vi "Main.vi"() -> ()   [LabVIEW 2013]
doc: "Use this template to build a producer/consumer design pattern with events to produce queue items. Use this design pattern instead of the User Interface Event Handler pattern for user interfaces when you want to execute code asynchronously in response to an event without slowing the user interface responsiveness."
uses:
  Controls.llb/ports_list.ctl
  Controls.llb/states.ctl
  Controls.llb/smu_2450_cmd.ctl
  Controls.llb/smu_2450_qry.ctl
  Clusters.llb/main_clstr.ctl
  <instrlib>/Keithley 3706/Keithley 3700 Series.lvlib
  <instrlib>/Keithley 2450 LabVIEW 8/Keithley 2450.lvlib
panel:
  in  "open_res":dbl=5000000.0 caption="Open Res Value (Ohm)" format="%^#_6g"
  in  "cPCI":bool
  in  "bob_156":bool
  in  "bob_78":bool
  in  "save_file_qry":bool caption="Save File?"
  in  "create_file":bool
  in  "config_smu_funct":u16(ring) caption="Measuring SMU Function" items=["Volts", "Current", "Auto Resistance", "Manual Resistance", "Digitize Voltage", "Digitize Current"]
  in  "config_src":u16(ring) caption="Config Driving Source" items=["Volts", "Current"]
  in  "src_mode":u16(ring) caption="Source Type" items=["Volts", "Current"]
  in  "src_level":dbl=0.01 caption="Source Level (V/A)"
  in  "src_lim":dbl=1.0 caption="Source Limit (V/A)"
  in  "config_meas_type":u16(ring) caption="Configure Meas Type" items=["Volts", "Current", "Resistance"]
  in  "enb_auto_range":bool=TRUE caption="Auto Range"
  in  "Manual Range (1.0)":dbl=1.0 caption="Manual Range"
  out "main_states_ind":T1 caption="Status"
  in  "cpci_bob":bool caption="cPCI or BOB"
  in  "map_path":path caption="Mapping File"
  in  "stop":bool
  in  "main_tab":T2(tab)
  in  "num_of_cycles":u32=10 caption="Number of Cycles"
  in  "cycle":bool
  in  "strt_meas":bool
  in  "Table Control":T3 caption="Measuring Ports"
  in  "dwell_ms":u32=2000 caption="Measurement Dwell (ms)"
  in  "current":dbl=4.9999999999999886e-06 caption="Enter the Current Source (A)" format="%_3p"
  in  "vlim":dbl=1.0 caption="Enter the Voltage Limit (V)" format="%_3p"
  out "cyc_cntr_ind":u32 caption="Cycle Counter"
  in  "config_meas_params":bool
  in  "read_smu_data":bool
  in  "close_port":bool
  in  "cls_chnl_list":string="11306,11411" caption="Close Channel List"
  in  "open_chnl_list":string="11306,11411" caption="Open Channel List"
  in  "open_port":bool
  in  "open_all":bool
  in  "cls_chnl_list_bkpln":string="11306,11411" caption="Backplane Channel List"
  in  "config_bkplane":bool
  in  "bkpl_relays":string="10914" caption="Backplane Relays"
  in  "close_list":string="allslots" caption="Close Channel List"
  in  "get_closed_list":bool
  out "closed_list":string caption="Closed List"
  in  "enb_out":bool=TRUE caption="Enable Source"
  out "smu_data":string caption="SMU DATA"
  out "res_val":dbl caption="Resistance (Ohm)"
  in  "command":T4 caption="Command to Set"
  in  "set_cmnd":bool
  in  "qry_cmd 2":T5 caption="Command to Query"
  in  "qry_cmd":bool
  out "resp":string caption="Query Response"
  in  "off_on":bool caption="OFF/ON"
  in  "smu_VISA_resource_name":refnum<visa-resource-name>="USBInstrument2" caption="SMU Visa Resource Name"
  in  "switch_VISA_resource_name":refnum<visa-resource-name>="USBInstrument3" caption="Switch Visa Resource Name"
  out "cpci_or_bob_table":string[][](array[string])
  out "port_list":string[][](array[string])
  in  "ports_path":path caption="Switching Ports File"
  in  "file_name_path":path=path "c:/data/test_one" caption="Enter File Name to Save (csv file)"
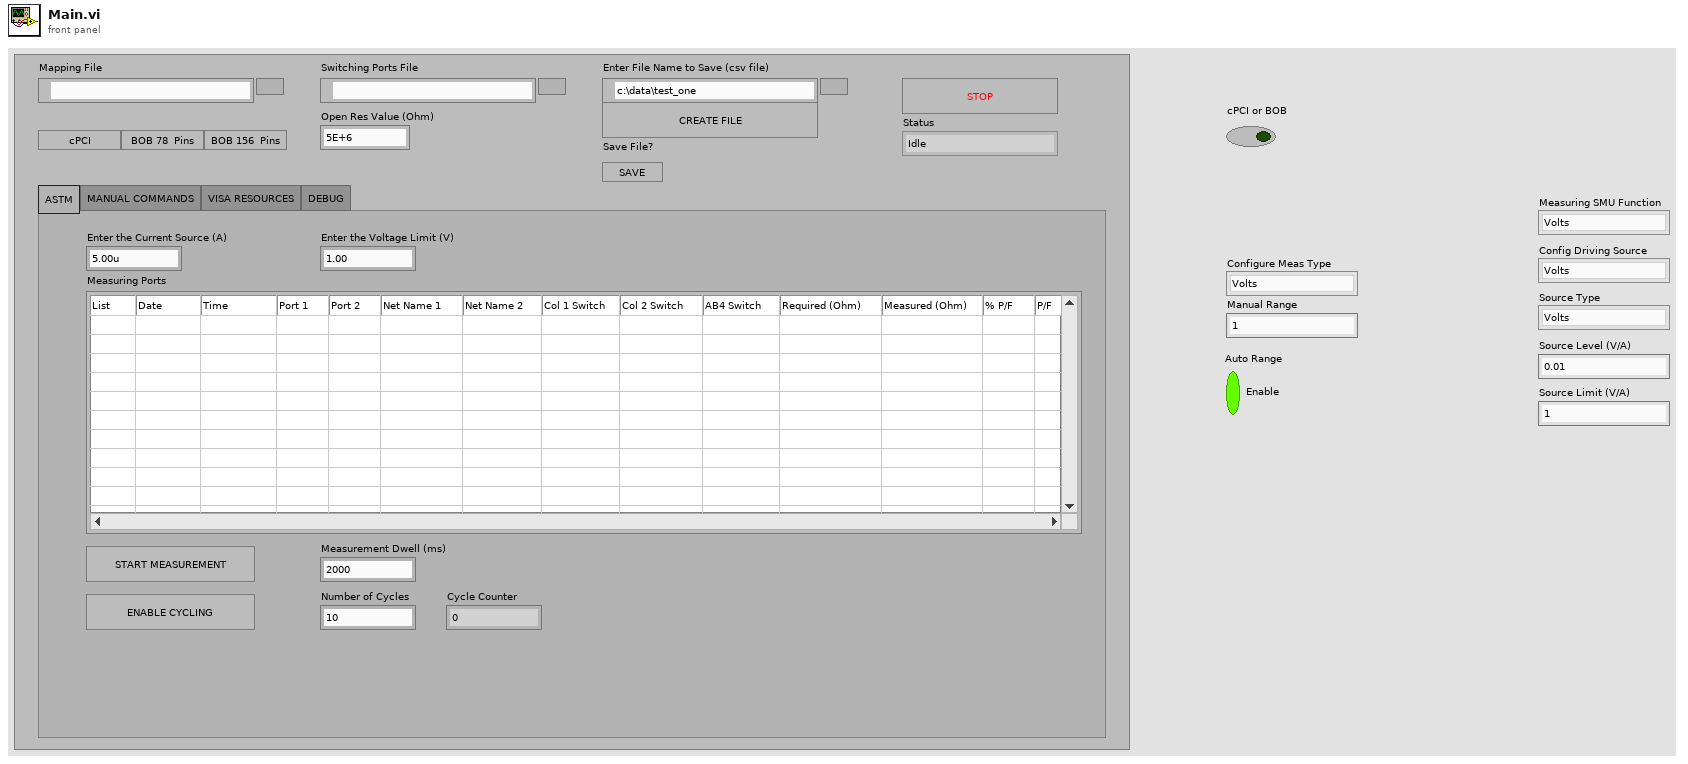
[diagram p1: front panel]
types:
  T1 = typedef "states.ctl" = enum16{"Idle", "Initalize", "Init Sec Visa", "Set_SMU_Current", "Check_for_1st_port", "Match_LUT", "Set_1st_port_flg", "1st_port_flg_chk", "2nd_port_flg_chk", "Clr_1st_port_flg", "Check_for_2nd_port", "Set_2nd_port_flg", "Clr_2nd_port_flg", "Finish_port_match_qry", "Nxt_port_meas_incr", "Enb_SMU", "Disable_SMU", "Close_ports", "Open_ports", "Take_Res_Meas", "Store_Res_Meas", "Comp_Res_Meas", "Disp_Meas", "Finish_Test_Qry", "Go_to_nxt_meas", "Search cPCI Pin", "Set Adj Col Pin", "Set Bank Number", "Pop Cons Data", "Select Adj Col Cnt", "Sel Slot Number", "Build 1st Port SBRCC Code", "Build 2nd Port SBRCC Code", "Set AB4 Code", "Make Meas", "Dwell", "Cycling_Qry", "Fin_Cyc_Qry", "Clr_Cyc_Cntr", "Test_Cancel_Qry", "Incr_cyc_cntr", "Clr_Table_Cols", "Incr_File_Name", "Save_File", "clr_queue"}
  T2 = enum32{"ASTM", "MANUAL COMMANDS", "VISA RESOURCES", "DEBUG"}
  T3 = typedef "ports_list.ctl" = string[][]
  T4 = typedef "smu_2450_cmd.ctl" = enum16{"Res_Sen", "Res_Comp"}
  T5 = typedef "smu_2450_qry.ctl" = enum16{"Res_Sen", "Res_Comp"}
  T6 = typedef "main_clstr.ctl" = cluster{"main_states":T1, "port_row":i32, "first_port_flg":bool, "first_port_arry":string[], "second_port_arry":string[], "first_port_col":string[], "second_port_col":string[], "second_port_flg":bool, "num_of_meas":i32, "sw_visa_res_out":refnum<visa-resource-name>, "map_table":string[][], "sw_pins":string[][], "port_indx_row":i32, "second_port_indx":i32, "adj_col_cnt":string, "bank_number":string, "row_number":string, "slot_number":string, "ab_code":string[], "Table Control":T3, "smu_visa_res_out":refnum<visa-resource-name>, "meas_res_str":string, "cyc_cntr":u32, "cyc_cntr_ind":u32, "file_name_incr":refnum<file>, "file_name_ref":refnum<file>}
  T7 = enum16{"open", "replace", "create", "open or create", "replace or create", "replace or create with confirmation"}
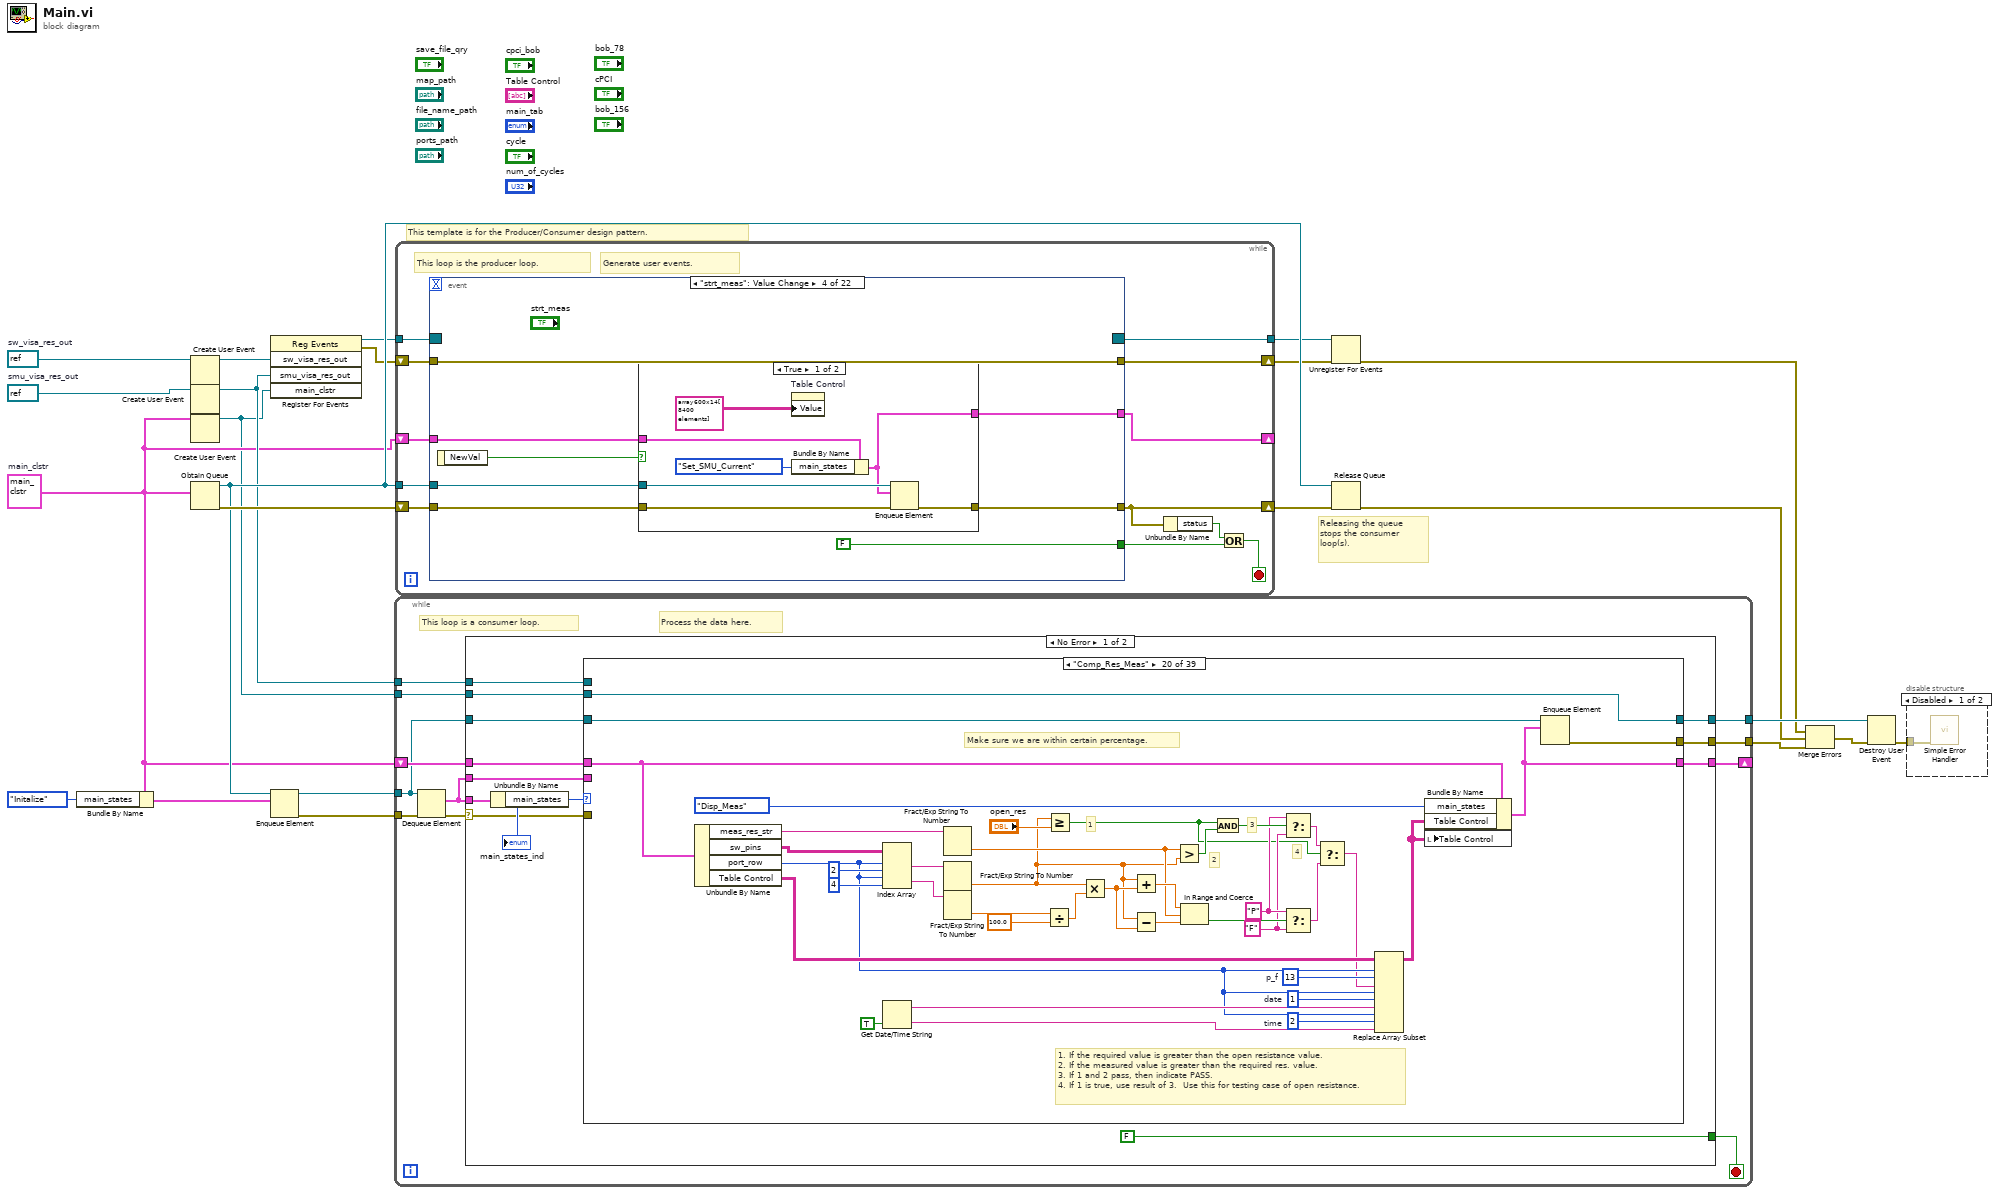
[diagram p0: block diagram]
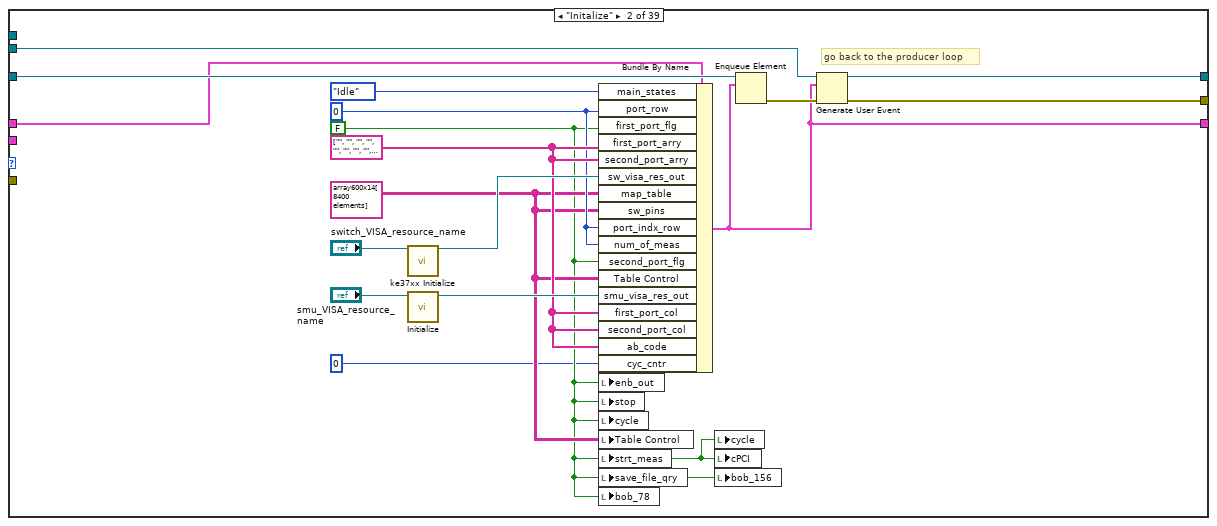
[diagram p4: hidden frame]
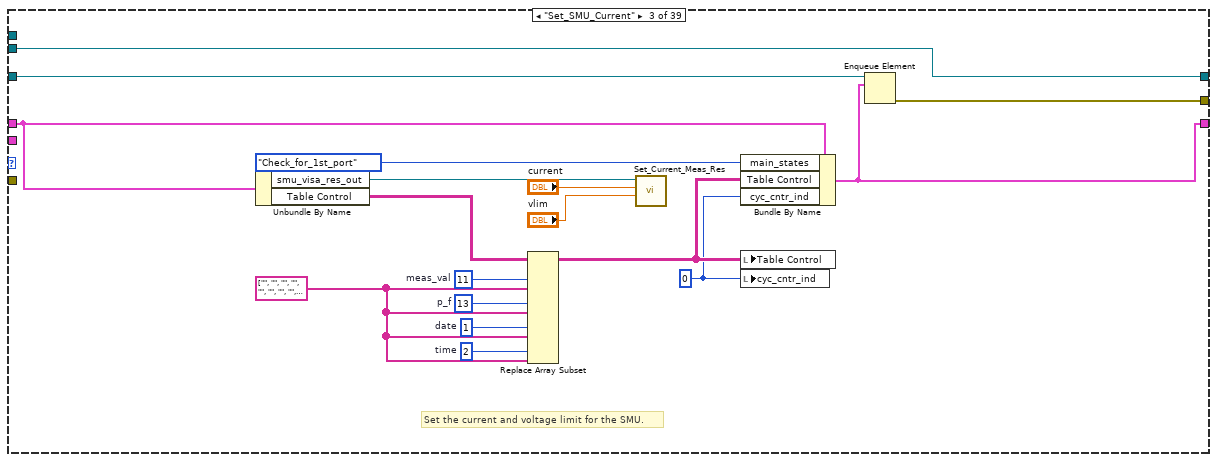
[diagram p5: hidden frame]
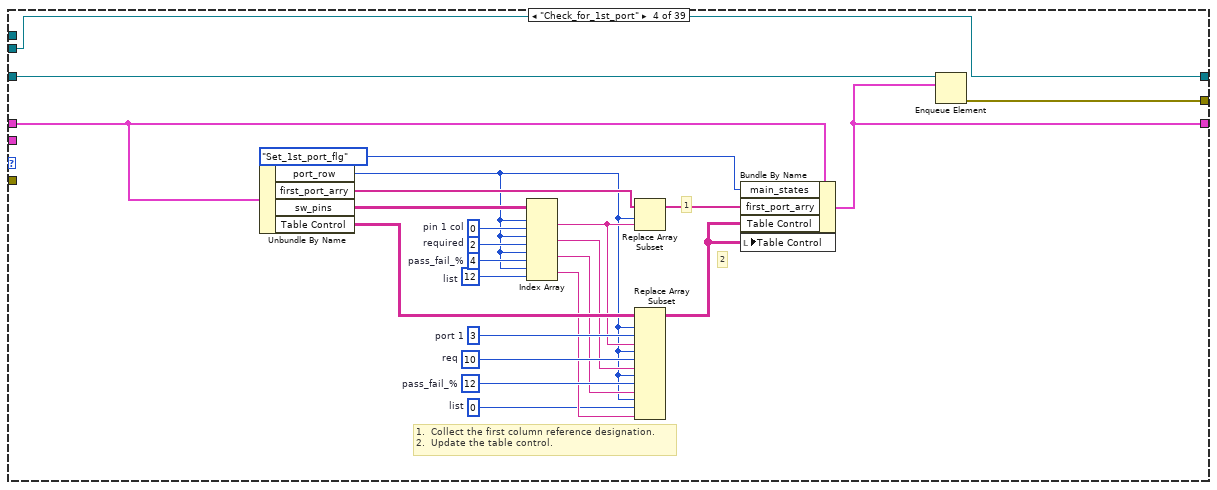
[diagram p6: hidden frame]
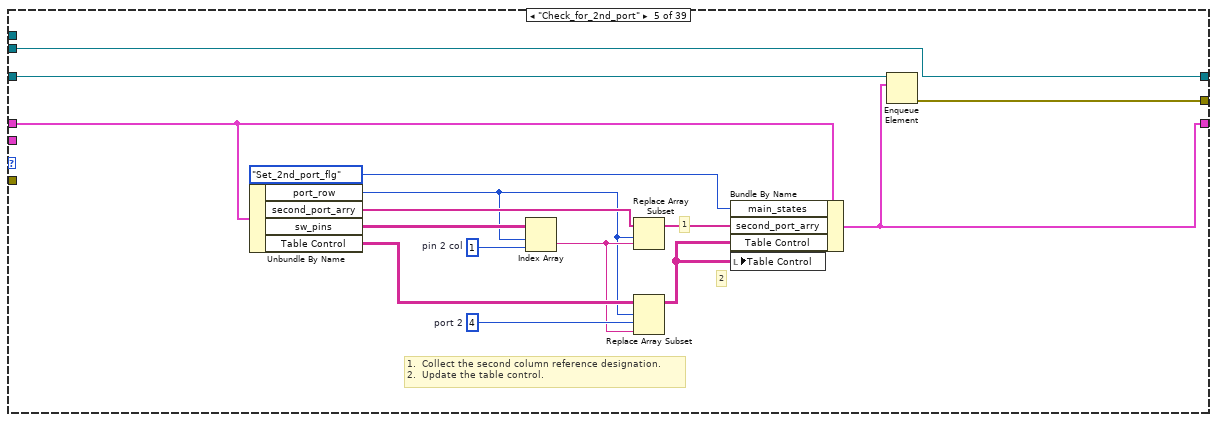
[diagram p7: hidden frame]
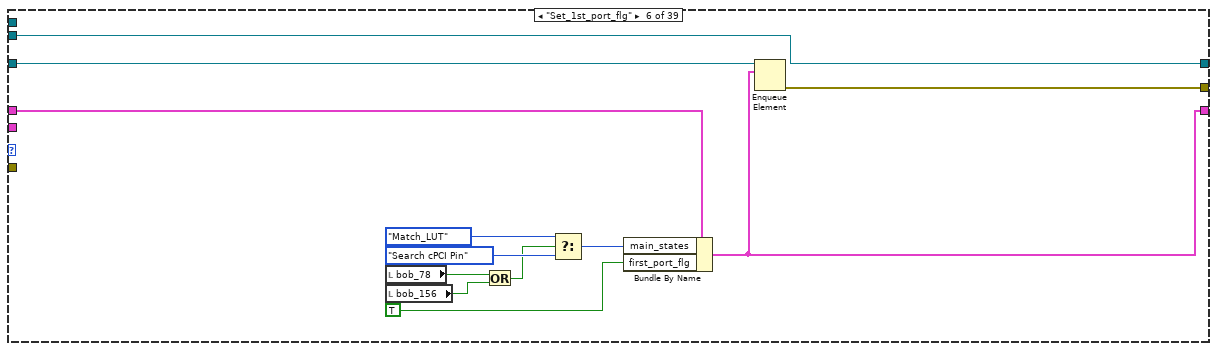
[diagram p8: hidden frame]
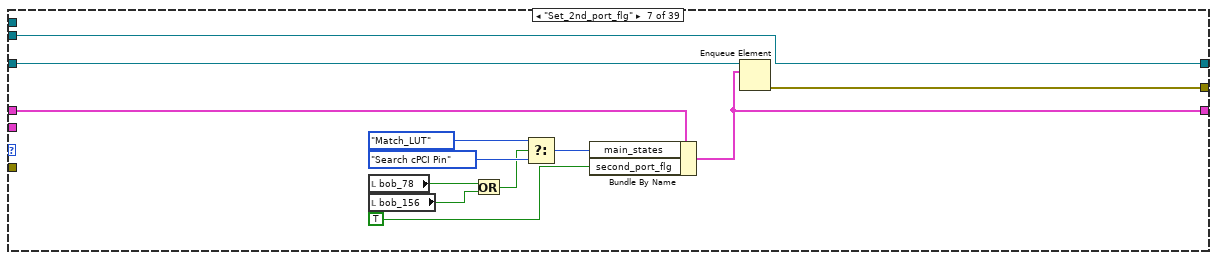
[diagram p9: hidden frame]
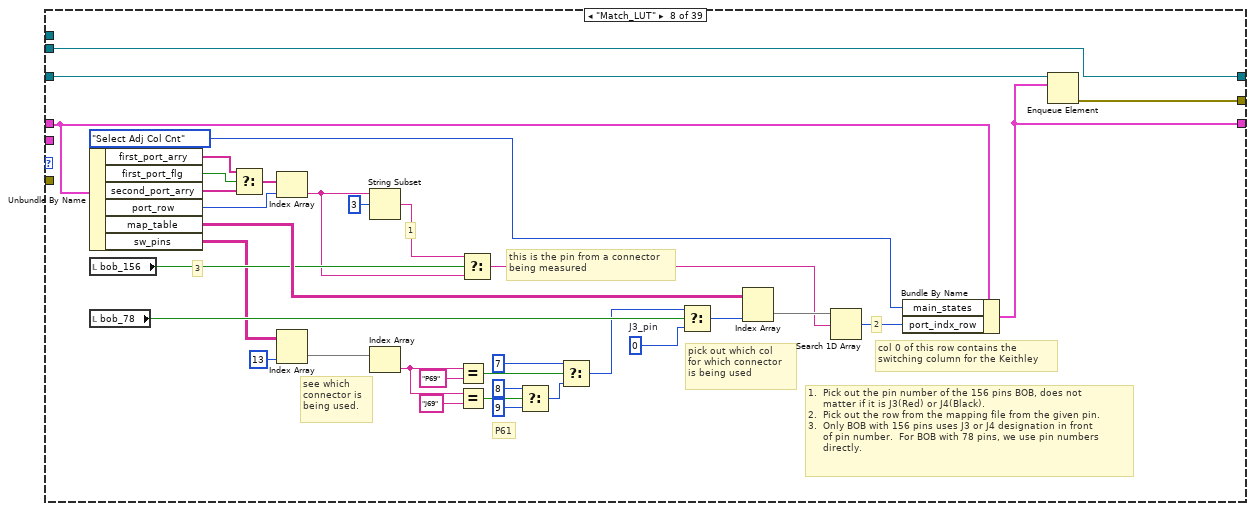
[diagram p10: hidden frame]
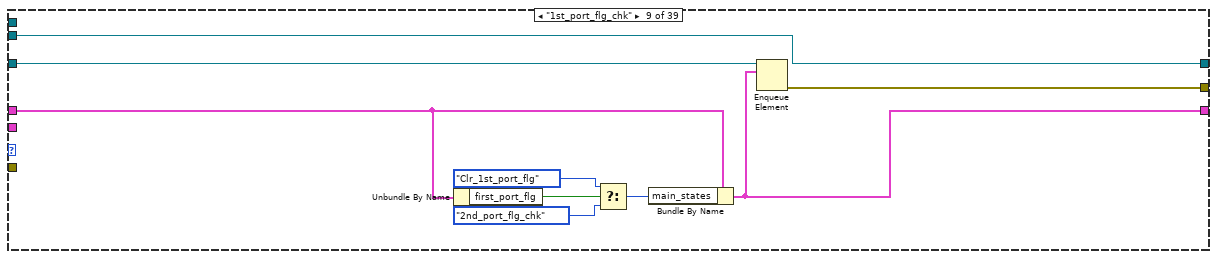
[diagram p11: hidden frame]
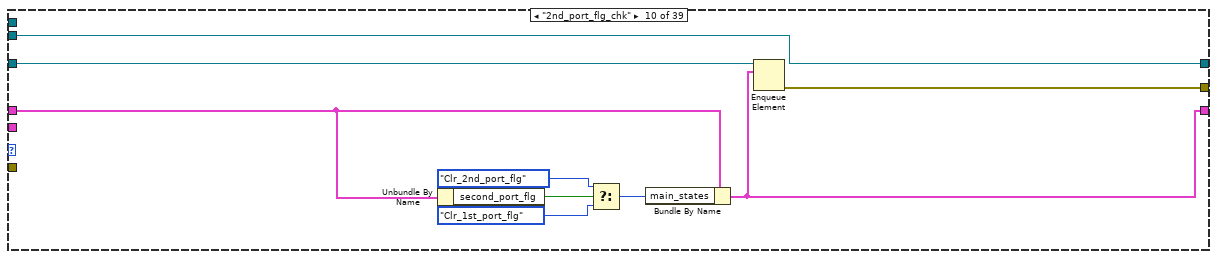
[diagram p12: hidden frame]
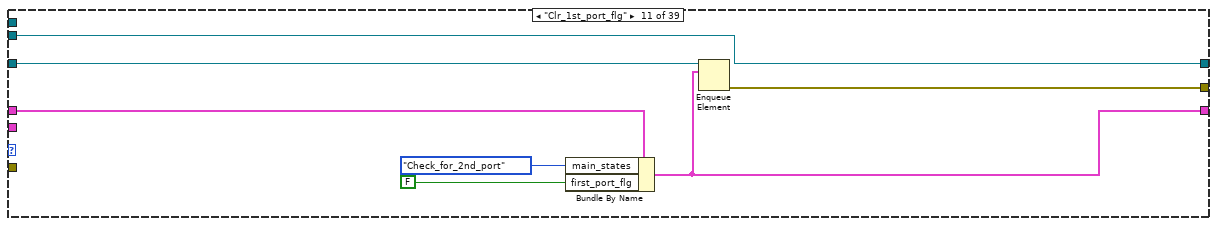
[diagram p13: hidden frame]
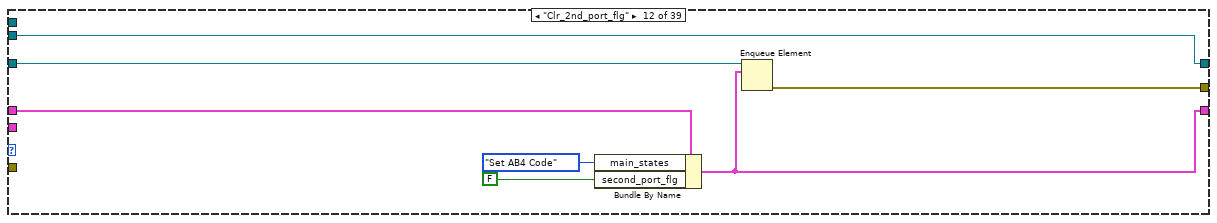
[diagram p14: hidden frame]
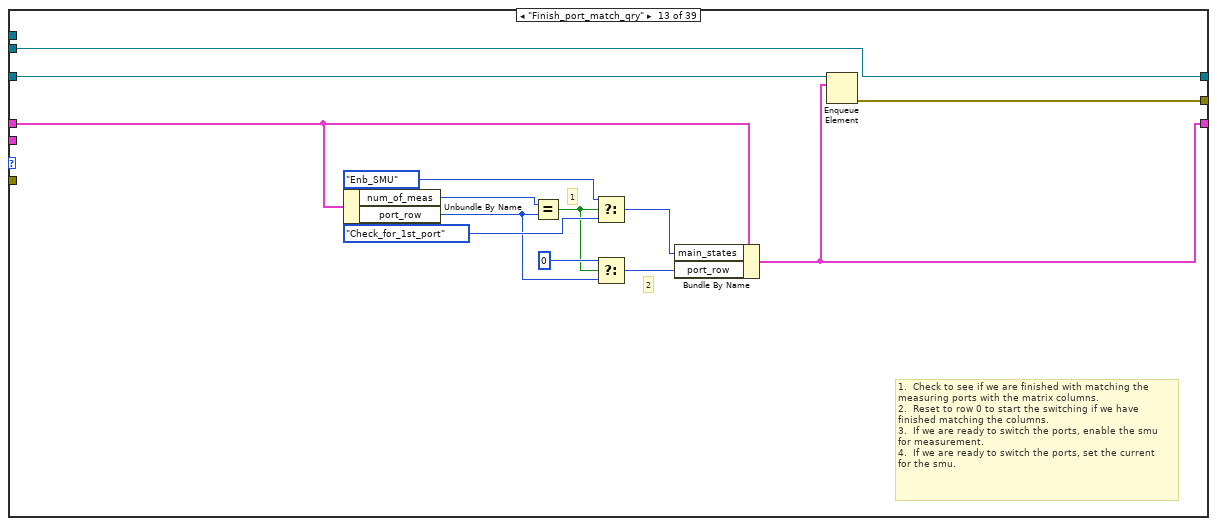
[diagram p15: hidden frame]
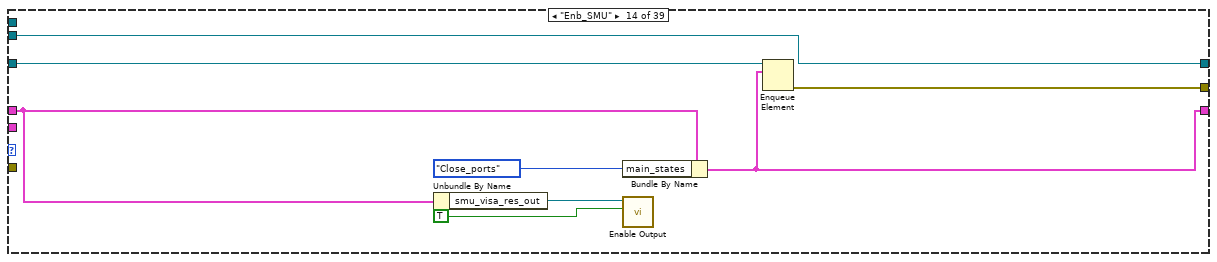
[diagram p16: hidden frame]
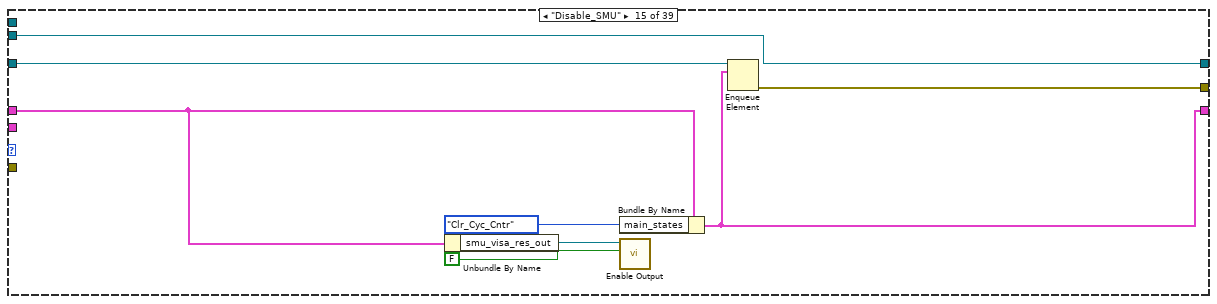
[diagram p17: hidden frame]
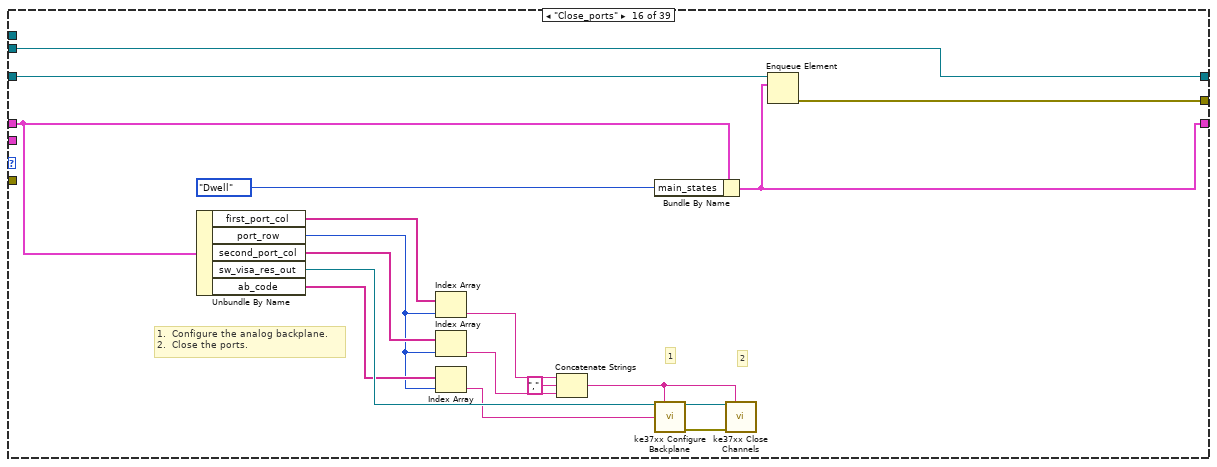
[diagram p18: hidden frame]
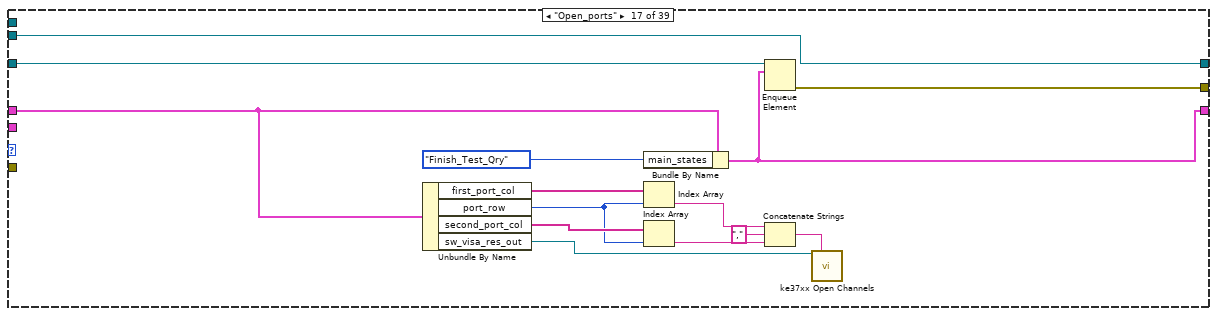
[diagram p19: hidden frame]
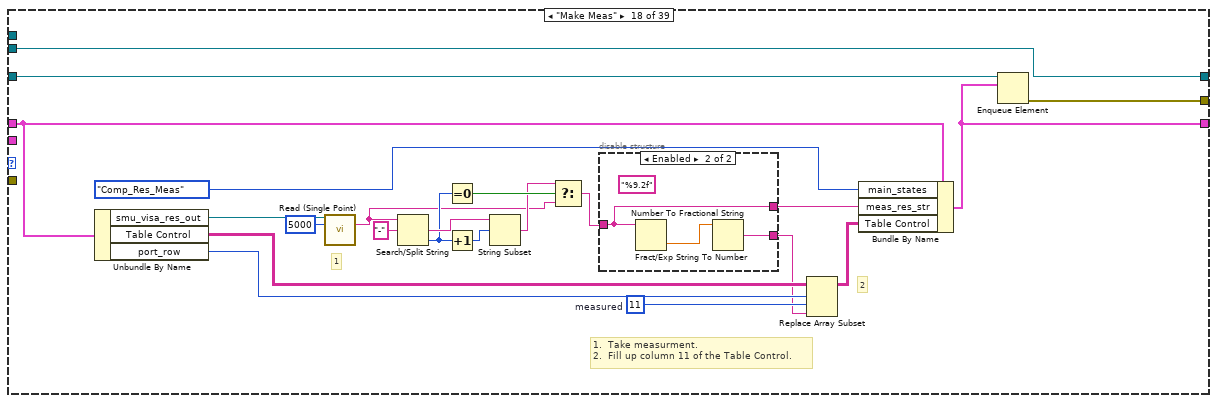
[diagram p20: hidden frame]
diagram:
  w5 = refnum<visa-resource-name> refnum  # smu_visa_res_out
  w9 = refnum<visa-resource-name> refnum  # sw_visa_res_out
  w2 = T6 {"main_states"=enum."Idle", "port_row"=0, "first_port_flg"=FALSE, "first_port_arry"=[], "second_port_arry"=[], "first_port_col"=[], "second_port_col"=[], "second_port_flg"=FALSE, "num_of_meas"=0, "sw_visa_res_out"="", "map_table"=[], "sw_pins"=[], "port_indx_row"=0, "second_port_indx"=0, "adj_col_cnt"="", "bank_number"="", "row_number"="", "slot_number"="", "ab_code"=[], "Table Control"=[], "smu_visa_res_out"="", "meas_res_str"="", "cyc_cntr"=0, "cyc_cntr_ind"=0, "file_name_incr"=refnum, "file_name_ref"=refnum}  # main_clstr
  # "Releasing the queue stops the consumer loop(s)."
  # "This template is for the Producer/Consumer design pattern."
  n1 = Bundle By Name(cluster=w2, "main_states"=states."Initalize") -> (w19:T6)
  n2 = Create User Event(user event datatype=w9) -> (user event=w10:refnum<user-event>)  [unwired: 1 in, 1 out]
  n3 = Create User Event(user event datatype=w5) -> (user event=w4:refnum<user-event>)  [unwired: 1 in, 1 out]
  n4 = Create User Event(user event datatype=w2) -> (user event=w1:refnum<user-event>)  [unwired: 1 in, 1 out]
  n5 = Obtain Queue(element data type=w2) -> (queue out=w21:refnum<queue>, error out=w23:errorcluster)  [unwired: 4 in, 1 out]
  n6 = register-events(w10, w4, w1) -> (reference out=w8:refnum<event-registration>, error out=w7:errorcluster)  [unwired: 2 in]
  n7 = Enqueue Element(queue=w21, element=w19) -> (queue out=w20:refnum<queue>, error out=w6:errorcluster)  [unwired: 2 in, 1 out]
  n8 = while {
    tunnel: w20 -> [w31]
    shift-right: [w32] -> _
    shift-left: w2 -> [w33]
    tunnel: w1 -> [w30]
    tunnel: [w29] -> w14
    tunnel: [w28] -> w13
    tunnel: w6 -> [w27]
    tunnel: w4 -> [w26]
    stop <- w24 stop-if-true
    # "Process the data here."
    # "This loop is a consumer loop."
    n9 = Dequeue Element(queue=w31, error in (no error)=w27) -> (element=w25:T6, error out=w34:errorcluster)  [unwired: 1 in, 2 out]
    n10 = case shown="No Error" w34 {
      selector: w34 -> [w37 w683]
      tunnel: w25 -> [w45 _]
      tunnel: [FALSE TRUE] -> w24
      tunnel: w33 -> [w43 w685]
      tunnel: [w42 w685] -> w32
      tunnel: w31 -> [w41 _]
      tunnel: w30 -> [w40 w684]
      tunnel: [w39 w684] -> w29
      tunnel: [w38 w683] -> w28
      tunnel: w26 -> [w36 _]
      tunnel: w25 -> [w35 _]
      frame No Error {
        n11 = Unbundle By Name(w45) -> ("main_states"=w44:T1)
        "main_states_ind" <- w44
        n12 = case shown="\"Comp_Res_Meas\"" w44 {
          tunnel: w43 -> [w49 w65 w79 w106 w110 w133 w135 w147 w185 w194 w205 w212 w221 w228 w236 w244 w273 w293 w304 w349 w354 w374 w398 w417 w427 w452 w495 w538 w555 w572 w588 w596 w619 w625 w640 w649 w664 w672 w682]
          tunnel: [w49 w55 w67 w84 w108 w123 w137 w149 w182 w191 w200 w207 w214 w227 w235 w243 w261 w284 w303 w325 w353 w363 w379 w403 w422 w432 w454 w497 w541 w557 w574 w591 w601 w624 w637 w644 w661 w670 w678] -> w42
          tunnel: w41 -> [_ w66 w83 w105 w121 w132 w146 w181 w190 w199 w206 w213 w226 w234 w242 w260 w274 w296 w307 w352 w359 w378 w402 w421 w430 w453 w496 w539 w556 w573 w589 w600 w623 w635 w643 w652 w667 w675 w681]
          tunnel: w40 -> [w48 w61 w82 w103 w119 w131 w145 w176 w183 w193 w203 w210 w223 w233 w241 w259 w272 w295 w306 w351 w358 w377 w401 w419 w429 w451 w494 w537 w554 w571 w587 w599 w622 w634 w642 w651 w666 w674 w680]
          tunnel: [w48 w59 w82 w103 w119 w131 w145 w176 w183 w193 w203 w210 w223 w233 w241 w259 w272 w295 w306 w351 w358 w377 w401 w419 w429 w451 w494 w537 w554 w571 w587 w599 w622 w634 w642 w651 w666 w674 w680] -> w39
          tunnel: [w47 w58 w81 w102 w118 w130 w144 w175 w184 w192 w202 w209 w222 w232 w240 w258 w271 w294 w305 w350 w357 w376 w400 w418 w428 w450 w493 w536 w553 w570 w586 w598 w621 w633 w641 w650 w665 w673 w679] -> w38
          tunnel: w37 -> [w47 _ _ _ _ _ _ _ _ _ _ _ _ _ _ _ _ _ _ _ _ _ _ _ _ _ _ _ _ _ _ _ _ _ _ _ _ _ _]
          tunnel: w36 -> [_ _ _ _ _ _ _ _ _ _ _ _ _ _ _ _ _ _ _ _ _ _ _ _ _ _ _ _ _ _ _ _ _ _ _ _ _ _ _]
          tunnel: w35 -> [_ _ _ _ _ _ _ _ _ _ _ _ _ _ _ _ _ _ _ _ _ _ _ _ _ _ _ _ _ _ _ w593 _ _ _ _ _ _ _]
          frame "Idle", Default {
          }
          frame "Initalize" {
            w52 = string[][] array600x14[8400 elements] ("cpci_table")
            w54 = string[] ["", "", "", "", "", "", "", "", "", "", "", "", "", "", "", "", "", "", "", "", "", "", "", "", "", "", "", "", "", "", "", "", "", "", "", "", "", "", "", "", "", "", "", "", "", "", "", "", "", "", "", "", "", "", "", "", "", "", "", "", "", "", "", "", "", "", "", "", "", "", "", "", "", "", "", "", "", "", "", "", "", "", "", "", "", "", "", "", "", "", "", "", "", "", "", "", "", "", "", "", "", "", "", "", "", "", "", "", "", "", "", "", "", "", "", "", "", "", "", "", "", "", "", "", "", "", "", "", "", "", "", "", "", "", "", "", "", "", "", "", "", "", "", "", "", "", "", "", "", "", "", "", "", "", "", "", "", "", "", "", "", "", "", "", "", "", "", "", "", "", "", "", "", "", "", "", "", "", "", "", "", "", "", "", "", "", "", "", "", "", "", "", "", "", "", "", "", "", "", "", "", "", "", "", "", "", "", "", "", "", "", "", "", "", "", "", "", "", "", "", "", "", "", "", "", "", "", "", "", "", "", "", "", "", "", "", "", "", "", "", "", "", "", "", "", "", "", "", "", "", "", "", "", "", "", "", "", "", "", "", "", "", "", "", "", "", "", "", "", "", "", "", "", "", "", "", "", "", "", "", "", "", "", "", "", "", "", "", "", "", "", "", "", "", "", "", "", "", "", "", "", "", "", "", "", "", "", "", "", "", "", "", "", "", "", "", "", "", "", "", "", "", "", "", "", "", "", "", "", "", "", "", "", "", "", "", "", "", "", "", "", "", "", "", "", "", "", "", "", "", "", "", "", "", "", "", "", "", "", "", "", "", "", "", "", "", "", "", "", "", "", "", "", "", "", "", "", "", "", "", "", "", "", "", "", "", "", "", "", "", "", "", "", "", "", "", "", "", "", "", "", "", "", "", "", "", "", "", "", "", "", "", "", "", "", "", "", "", "", "", "", "", "", "", "", "", "", "", "", "", "", "", "", "", "", "", "", "", "", "", "", "", "", "", "", "", "", "", "", "", "", "", "", "", "", "", "", "", "", "", "", "", "", "", "", "", "", "", "", "", "", "", "", "", "", "", "", "", "", "", "", "", "", "", "", "", "", "", "", "", "", "", "", "", "", "", "", "", "", "", " ", "", "", "", "", "", "", "", "", "", "", "", "", "", "", "", "", "", "", "", "", "", "", "", "", "", "", "", "", "", "", "", "", "", "", "", "", "", "", "", "", "", "", "", "", "", "", "", "", "", "", "", "", "", "", "", "", "", "", "", "", "", "", "", "", "", "", "", "", "", "", "", "", "", "", "", "", "", "", "", "", "", "", "", "", "", "", "", "", "", "", "", "", "", "", "", "", "", "", " "] ("first_port_str")
            w51 = FALSE ("first_port_flg")
            w53 = 0 ("port_row")
            # "go back to the producer loop"
            n13 = call <instrlib>:"ke37xx Initialize.vi"("VISA resource name"="switch_VISA_resource_name") -> ("VISA resource name out"=w60:refnum<visa-resource-name>)  [unwired: 13 in, 1 out]
            n14 = call <instrlib>:"Initialize.vi"("VISA resource name"="smu_VISA_resource_name") -> ("VISA resource name out"=w56:refnum<visa-resource-name>)  [unwired: 9 in, 1 out]
            n15 = Bundle By Name(cluster=w65, "main_states"=states."Idle", "port_row"=w53, "first_port_flg"=w51, "first_port_arry"=w54, "second_port_arry"=w54, "sw_visa_res_out"=w60, "map_table"=w52, "sw_pins"=w52, "port_indx_row"=w53, "num_of_meas"=w53, "second_port_flg"=w51, "Table Control"=w52, "smu_visa_res_out"=w56, "first_port_col"=w54, "second_port_col"=w54, "ab_code"=w54, "cyc_cntr"=u32 0) -> (w55:T6)
            n16 = local write "enb_out"(w51) -> ()
            n17 = local write "stop"(w51) -> ()
            n18 = local write "cycle"(w51) -> ()
            n19 = local write "Table Control"(w52) -> ()
            n20 = local write "strt_meas"(w51) -> ()
            n21 = local write "save_file_qry"(w51) -> ()
            n22 = local write "bob_78"(w51) -> ()
            n23 = local write "cycle"(w51) -> ()
            n24 = local write "cPCI"(w51) -> ()
            n25 = local write "bob_156"(w51) -> ()
            n26 = Enqueue Element(queue=w66, element=w55) -> (error out=w62:errorcluster)  [unwired: 2 in, 2 out]
            n27 = Generate User Event(user event=w61, event data cluster=w55, error in=w62) -> (user event out=w59:refnum<user-event>, error out=w58:errorcluster)  [unwired: 1 in]
          }
          frame "Set_SMU_Current" {
            w70 = 2  # time
            w71 = 1  # date
            w72 = u32 0 ("cyc_cntr_ind")
            w74 = 13  # p_f
            w69 = string[] ["", "", "", "", "", "", "", "", "", "", "", "", "", "", "", "", "", "", "", "", "", "", "", "", "", "", "", "", "", "", "", "", "", "", "", "", "", "", "", "", "", "", "", "", "", "", "", "", "", "", "", "", "", "", "", "", "", "", "", "", "", "", "", "", "", "", "", "", "", "", "", "", "", "", "", "", "", "", "", "", "", "", "", "", "", "", "", "", "", "", "", "", "", "", "", "", "", "", "", "", "", "", "", "", "", "", "", "", "", "", "", "", "", "", "", "", "", "", "", "", "", "", "", "", "", "", "", "", "", "", "", "", "", "", "", "", "", "", "", "", "", "", "", "", "", "", "", "", "", "", "", "", "", "", "", "", "", "", "", "", "", "", "", "", "", "", "", "", "", "", "", "", "", "", "", "", "", "", "", "", "", "", "", "", "", "", "", "", "", "", "", "", "", "", "", "", "", "", "", "", "", "", "", "", "", "", "", "", "", "", "", "", "", "", "", "", "", "", "", "", "", "", "", "", "", "", "", "", "", "", "", "", "", "", "", "", "", "", "", "", "", "", "", "", "", "", "", "", "", "", "", "", "", "", "", "", "", "", "", "", "", "", "", "", "", "", "", "", "", "", "", "", "", "", "", "", "", "", "", "", "", "", "", "", "", "", "", "", "", "", "", "", "", "", "", "", "", "", "", "", "", "", "", "", "", "", "", "", "", "", "", "", "", "", "", "", "", "", "", "", "", "", "", "", "", "", "", "", "", "", "", "", "", "", "", "", "", "", "", "", "", "", "", "", "", "", "", "", "", "", "", "", "", "", "", "", "", "", "", "", "", "", "", "", "", "", "", "", "", "", "", "", "", "", "", "", "", "", "", "", "", "", "", "", "", "", "", "", "", "", "", "", "", "", "", "", "", "", "", "", "", "", "", "", "", "", "", "", "", "", "", "", "", "", "", "", "", "", "", "", "", "", "", "", "", "", "", "", "", "", "", "", "", "", "", "", "", "", "", "", "", "", "", "", "", "", "", "", "", "", "", "", "", "", "", "", "", "", "", "", "", "", "", "", "", "", "", "", "", "", "", "", "", "", "", "", "", "", "", "", "", "", "", "", "", "", "", "", "", "", "", "", "", "", "", "", "", "", "", "", "", "", "", "", "", "", "", "", "", "", "", "", "", "", "", "", "", "", "", "", "", "", "", "", "", "", "", "", "", "", "", "", "", "", "", "", "", "", "", "", "", "", "", "", "", "", "", "", "", "", "", "", "", "", "", "", "", "", "", "", "", "", "", "", "", "", "", "", "", "", "", "", "", "", "", "", "", "", "", "", "", "", "", "", "", "", "", "", "", "", "", "", "", "", "", "", "", "", "", " "] ("new element/subarray")
            w76 = 11  # meas_val
            # "Set the current and voltage limit for the SMU."
            n28 = Unbundle By Name(w79) -> ("smu_visa_res_out"=w80:refnum<visa-resource-name>, "Table Control"=w73:T3)
            n29 = Replace Array Subset(array=w73, new element #1=w69, index (col) #1=w76, new element #2=w69, index (col) #2=w74, new element #3=w69, index (col) #3=w71, new element #4=w69, index (col) #4=w70) -> (w75:T3)  [unwired: 4 in]
            n30 = call "Set_Current_Meas_Res.vi"("vlim"="vlim", "current"="current", "VISA resource name"=w80) -> ()  [unwired: 8 in, 1 out]
            n31 = Bundle By Name(cluster=w79, "main_states"=states."Check_for_1st_port", "Table Control"=w75, "cyc_cntr_ind"=w72) -> (w67:T6)
            n32 = local write "Table Control"(w75) -> ()
            n33 = local write "cyc_cntr_ind"(w72) -> ()
            n34 = Enqueue Element(queue=w83, element=w67) -> (error out=w81:errorcluster)  [unwired: 2 in, 2 out]
          }
          frame "Check_for_1st_port" {
            w86 = 0  # list
            w89 = 12  # list
            w91 = 12  # pass_fail_%
            w93 = 10  # req
            w94 = 4  # pass_fail_%
            w95 = 2  # required
            w99 = 3  # port 1
            w107 = 0  # pin 1 col
            # "2"
            # "1"
            # "1.  Collect the first column reference designation.\n2.  Update the table control."
            n35 = Unbundle By Name(w106) -> ("port_row"=w87:i32, "first_port_arry"=w98:string[], "sw_pins"=w101:string[][], "Table Control"=w100:T3)
            n36 = Index Array(array=w101, index (row) #1=w87, index (col) #1=w107, index (row) #2=w87, index (col) #2=w95, index (row) #3=w87, index (col) #3=w94, index (row) #4=w87, index (col) #4=w89) -> (element #1=w96:string, element #2=w92:string, element #3=w90:string, element #4=w88:string)
            n37 = Replace Array Subset(array=w98, new element=w96, index=w87) -> (w104:string[])
            n38 = Replace Array Subset(array=w100, new element #1=w96, index (row) #1=w87, index (col) #1=w99, new element #2=w92, index (row) #2=w87, index (col) #2=w93, new element #3=w90, index (row) #3=w87, index (col) #3=w91, new element #4=w88, index (row) #4=w87, index (col) #4=w86) -> (w97:T3)
            n39 = Bundle By Name(cluster=w106, "main_states"=states."Set_1st_port_flg", "first_port_arry"=w104, "Table Control"=w97) -> (w84:T6)
            n40 = local write "Table Control"(w97) -> ()
            n41 = Enqueue Element(queue=w105, element=w84) -> (error out=w102:errorcluster)  [unwired: 2 in, 2 out]
          }
          frame "Check_for_2nd_port" {
            w115 = 4  # port 2
            w122 = 1  # pin 2 col
            # "2"
            # "1"
            # "1.  Collect the second column reference designation.\n2.  Update the table control."
            n42 = Unbundle By Name(w110) -> ("port_row"=w111:i32, "second_port_arry"=w114:string[], "sw_pins"=w117:string[][], "Table Control"=w116:T3)
            n43 = Index Array(array=w117, index (row)=w111, index (col)=w122) -> (element=w112:string)
            n44 = Replace Array Subset(array=w114, new element=w112, index=w111) -> (w120:string[])
            n45 = Replace Array Subset(array=w116, new element=w112, index (row)=w111, index (col)=w115) -> (w113:T3)
            n46 = Bundle By Name(cluster=w110, "main_states"=states."Set_2nd_port_flg", "second_port_arry"=w120, "Table Control"=w113) -> (w108:T6)
            n47 = local write "Table Control"(w113) -> ()
            n48 = Enqueue Element(queue=w121, element=w108) -> (error out=w118:errorcluster)  [unwired: 2 in, 2 out]
          }
          frame "Set_1st_port_flg" {
            n49 = local read "bob_78"() -> (w127:bool)
            n50 = local read "bob_156"() -> (w126:bool)
            n51 = Or(x=w127, y=w126) -> (x .or. y?=w125:bool)
            n52 = Select(t=states."Match_LUT" ("main_states"), s=w125, f=states."Search cPCI Pin" ("main_states")) -> (s? t:f=w124:T1)
            n53 = Bundle By Name(cluster=w133, "main_states"=w124, "first_port_flg"=TRUE) -> (w123:T6)
            n54 = Enqueue Element(queue=w132, element=w123) -> (error out=w130:errorcluster)  [unwired: 2 in, 2 out]
          }
          frame "Set_2nd_port_flg" {
            n55 = local read "bob_78"() -> (w140:bool)
            n56 = local read "bob_156"() -> (w139:bool)
            n57 = Or(x=w140, y=w139) -> (x .or. y?=w138:bool)
            n58 = Select(t=states."Match_LUT" ("main_states"), s=w138, f=states."Search cPCI Pin" ("main_states")) -> (s? t:f=w141:T1)
            n59 = Bundle By Name(cluster=w135, "main_states"=w141, "second_port_flg"=TRUE ("first_port_flg")) -> (w137:T6)
            n60 = Enqueue Element(queue=w146, element=w137) -> (error out=w144:errorcluster)  [unwired: 2 in, 2 out]
          }
          frame "Match_LUT" {
            w164 = 0  # J3_pin
            # "this is the pin from a connector\nbeing measured"
            # "col 0 of this row contains the\nswitching column for the Keithley"
            # "1.  Pick out the pin number of the 156 pins BOB, does not\n     matter if it is J3(Red) or J4(Black).\n2.  Pick out the row from the mapping file from the given pin.\n3.  Only BOB with 156 pins uses J3 or J4 designation in front\n     of pin number.  For BOB with 78 pins, we use pin numbers\n     directly."
            # "pick out which col\nfor which connector\nis being used"
            # "P61"
            # "see which\nconnector is \nbeing used."
            # "3"
            # "2"
            # "1"
            n61 = Unbundle By Name(w147) -> ("first_port_arry"=w180:string[], "first_port_flg"=w173:bool, "second_port_arry"=w179:string[], "port_row"=w177:i32, "map_table"=w174:string[][], "sw_pins"=w162:string[][])
            n62 = local read "bob_156"() -> (w169:bool)
            n63 = local read "bob_78"() -> (w167:bool)
            n64 = Select(t=w180, s=w173, f=w179) -> (s? t:f=w178:string[])
            n65 = Index Array(array=w178, index=w177) -> (element=w166:string)
            n66 = Index Array(array=w162, index (col)=13 ("disabled index (col)")) -> (element=w160:string[])  [unwired: 1 in]
            n67 = String Subset(string=w166, offset (0)=3) -> (substring=w168:string)  [unwired: 1 in]
            n68 = Index Array(array=w160) -> (element=w157:string)  [unwired: 1 in]
            n69 = Equal?(x=w157, y="P69") -> (x = y?=w156:bool)
            n70 = Equal?(x=w157, y="J69") -> (x = y?=w154:bool)
            n71 = Select(t=w168, s=w169, f=w166) -> (s? t:f=w165:string)
            n72 = Select(t=8, s=w154, f=9) -> (s? t:f=w151:i32)
            n73 = Select(t=7, s=w156, f=w151) -> (s? t:f=w150:i32)
            n74 = Select(t=w150, s=w167, f=w164) -> (s? t:f=w163:i32)
            n75 = Index Array(array=w174, index (col)=w163) -> (element=w171:string[])  [unwired: 1 in]
            n76 = Search 1D Array(1D array=w171, element=w165) -> (index of element=w170:i32)  [unwired: 1 in]
            n77 = Bundle By Name(cluster=w147, "main_states"=states."Select Adj Col Cnt", "port_indx_row"=w170) -> (w149:T6)
            n78 = Enqueue Element(queue=w181, element=w149) -> (error out=w175:errorcluster)  [unwired: 2 in, 2 out]
          }
          frame "1st_port_flg_chk" {
            n79 = Unbundle By Name(w185) -> ("first_port_flg"=w189:bool)
            n80 = Select(t=states."Clr_1st_port_flg" ("main_states"), s=w189, f=states."2nd_port_flg_chk" ("main_states")) -> (s? t:f=w186:T1)
            n81 = Bundle By Name(cluster=w185, "main_states"=w186) -> (w182:T6)
            n82 = Enqueue Element(queue=w190, element=w182) -> (error out=w184:errorcluster)  [unwired: 2 in, 2 out]
          }
          frame "2nd_port_flg_chk" {
            n83 = Unbundle By Name(w194) -> ("second_port_flg"=w198:bool)
            n84 = Select(t=states."Clr_2nd_port_flg" ("main_states"), s=w198, f=states."Clr_1st_port_flg" ("main_states")) -> (s? t:f=w195:T1)
            n85 = Bundle By Name(cluster=w194, "main_states"=w195) -> (w191:T6)
            n86 = Enqueue Element(queue=w199, element=w191) -> (error out=w192:errorcluster)  [unwired: 2 in, 2 out]
          }
          frame "Clr_1st_port_flg" {
            n87 = Bundle By Name(cluster=w205, "main_states"=states."Check_for_2nd_port", "first_port_flg"=FALSE) -> (w200:T6)
            n88 = Enqueue Element(queue=w206, element=w200) -> (error out=w202:errorcluster)  [unwired: 2 in, 2 out]
          }
          frame "Clr_2nd_port_flg" {
            n89 = Bundle By Name(cluster=w212, "main_states"=states."Set AB4 Code" ("f"), "second_port_flg"=FALSE ("first_port_flg")) -> (w207:T6)
            n90 = Enqueue Element(queue=w213, element=w207) -> (error out=w209:errorcluster)  [unwired: 2 in, 2 out]
          }
          frame "Finish_port_match_qry" {
            # "2"
            # "1"
            # "1.  Check to see if we are finished with matching the\nmeasuring ports with the matrix columns.\n2.  Reset to row 0 to start the switching if we have\nfinished matching the columns.\n3.  If we are ready to switch the ports, enable the smu\nfor measurement.\n4.  If we are ready to switch the ports, set the current\nfor the smu."
            n91 = Unbundle By Name(w221) -> ("num_of_meas"=w216:i32, "port_row"=w220:i32)
            n92 = Equal?(x=w216, y=w220) -> (x = y?=w217:bool)
            n93 = Select(t=states."Enb_SMU" ("main_states"), s=w217, f=states."Check_for_1st_port" ("main_states")) -> (s? t:f=w215:T1)
            n94 = Select(t=0, s=w217, f=w220) -> (s? t:f=w218:i32)
            n95 = Bundle By Name(cluster=w221, "main_states"=w215, "port_row"=w218) -> (w214:T6)
            n96 = Enqueue Element(queue=w226, element=w214) -> (error out=w222:errorcluster)  [unwired: 2 in, 2 out]
          }
          frame "Enb_SMU" {
            n97 = Unbundle By Name(w228) -> ("smu_visa_res_out"=w230:refnum<visa-resource-name>)
            n98 = Bundle By Name(cluster=w228, "main_states"=states."Close_ports") -> (w227:T6)
            n99 = call <instrlib>:"Enable Output.vi"("Enable Output (T: Enable)"=TRUE, "VISA resource name"=w230) -> ()  [unwired: 8 in, 2 out]
            n100 = Enqueue Element(queue=w234, element=w227) -> (error out=w232:errorcluster)  [unwired: 2 in, 2 out]
          }
          frame "Disable_SMU" {
            n101 = Unbundle By Name(w236) -> ("smu_visa_res_out"=w238:refnum<visa-resource-name>)
            n102 = Bundle By Name(cluster=w236, "main_states"=states."Clr_Cyc_Cntr") -> (w235:T6)
            n103 = call <instrlib>:"Enable Output.vi"("Enable Output (T: Enable)"=FALSE, "VISA resource name"=w238) -> ()  [unwired: 8 in, 2 out]
            n104 = Enqueue Element(queue=w242, element=w235) -> (error out=w240:errorcluster)  [unwired: 2 in, 2 out]
          }
          frame "Close_ports" {
            # "1.  Configure the analog backplane.\n2.  Close the ports."
            # "2"
            # "1"
            n105 = Unbundle By Name(w244) -> ("first_port_col"=w257:string[], "port_row"=w249:i32, "second_port_col"=w253:string[], "sw_visa_res_out"=w254:refnum<visa-resource-name>, "ab_code"=w250:string[])
            n106 = Index Array(array=w257, index=w249) -> (element=w251:string)
            n107 = Index Array(array=w253, index=w249) -> (element=w252:string)
            n108 = Index Array(array=w250, index=w249) -> (element=w248:string)
            n109 = Concatenate Strings(w251, "," ("string"), w252) -> (w255:string)
            n110 = Bundle By Name(cluster=w244, "main_states"=states."Dwell" ("f")) -> (w243:T6)
            n111 = call <instrlib>:"ke37xx Configure Backplane.vi"("VISA Resource Name"=w254, "Channel List"=w255, "Backplane Relays"=w248) -> ("VISA Resource Name Out"=w246:refnum<visa-resource-name>, "error out"=w245:errorcluster)  [unwired: 11 in]
            n112 = call <instrlib>:"ke37xx Close Channels.vi"("VISA Resource Name"=w246, "Channel List"=w255, "error in (no error)"=w245) -> ()  [unwired: 11 in, 2 out]
            n113 = Enqueue Element(queue=w260, element=w243) -> (error out=w258:errorcluster)  [unwired: 2 in, 2 out]
          }
          frame "Open_ports" {
            n114 = Unbundle By Name(w273) -> ("first_port_col"=w270:string[], "port_row"=w265:i32, "second_port_col"=w268:string[], "sw_visa_res_out"=w263:refnum<visa-resource-name>)
            n115 = Bundle By Name(cluster=w273, "main_states"=states."Finish_Test_Qry" ("f")) -> (w261:T6)
            n116 = Index Array(array=w270, index=w265) -> (element=w266:string)
            n117 = Index Array(array=w268, index=w265) -> (element=w267:string)
            n118 = Enqueue Element(queue=w274, element=w261) -> (error out=w271:errorcluster)  [unwired: 2 in, 2 out]
            n119 = Concatenate Strings(w266, "," ("string"), w267) -> (w262:string)
            n120 = call <instrlib>:"ke37xx Open Channels.vi"("VISA Resource Name"=w263, "Channel List"=w262) -> ()  [unwired: 12 in, 2 out]
          }
          frame "Make Meas" {
            w289 = 11  # measured
            # "2"
            # "1"
            # "1.  Take measurment.\n2.  Fill up column 11 of the Table Control."
            n121 = Unbundle By Name(w293) -> ("smu_visa_res_out"=w292:refnum<visa-resource-name>, "Table Control"=w291:T3, "port_row"=w290:i32)
            n122 = call <instrlib>:"Read (Single Point).vi"("VISA resource name"=w292, "Timeout (10000 ms)"=5000) -> ("Data out"=w277:string)  [unwired: 11 in, 2 out]
            n123 = Search/Split String(string=w277, search string/char (-)="-") -> (match + rest of string=w282:string, offset of match=w280:i32)  [unwired: 1 in, 1 out]
            n124 = Equal To 0?(x=w280) -> (x = 0?=w279:bool)
            n125 = Increment(x=w280) -> (x+1=w281:i32)
            n126 = String Subset(string=w282, offset (0)=w281) -> (substring=w278:string)  [unwired: 1 in]
            n127 = Select(t=w278, s=w279, f=w277) -> (s? t:f=w276:string)
            n128 = disable-structure shown="Enabled" {
              disable-tunnel: w276 -> [w299 w301]
              disable-tunnel: [w297 w301] -> w288
              disable-tunnel: [_ w300] -> w275
              frame Disabled {
                n129 = Format Into String(format string="%9.2s", w299) -> (resulting string=w297:string)  [unwired: 2 in, 1 out]
              }
              frame Enabled {
                (unwired) "%9.2f" ("format string")
                n130 = Fract/Exp String To Number(string=w301) -> (number=w302:dbl)  [unwired: 3 in, 1 out]
                n131 = Number To Fractional String(number=w302) -> (F-format string=w300:string)  [unwired: 3 in]
              }
            }
            n132 = Replace Array Subset(array=w291, new element=w275, index (row)=w290, index (col)=w289) -> (w287:T3)
            n133 = Bundle By Name(cluster=w293, "main_states"=states."Comp_Res_Meas", "meas_res_str"=w288, "Table Control"=w287) -> (w284:T6)
            n134 = Enqueue Element(queue=w296, element=w284) -> (error out=w294:errorcluster)  [unwired: 2 in, 2 out]
          }
          frame "Dwell" {
            n135 = stacked-sequence {
              tunnel: w307 -> [_ w313]
              tunnel: [_ w312] -> w305
              tunnel: w304 -> [_ w310]
              tunnel: [_ w309] -> w303
              frame #0 {
                n136 = Wait (ms)(milliseconds to wait="dwell_ms") -> ()  [unwired: 1 out]
              }
              frame #1 {
                n137 = Bundle By Name(cluster=w310, "main_states"=states."Make Meas") -> (w309:T6)
                n138 = Enqueue Element(queue=w313, element=w309) -> (error out=w312:errorcluster)  [unwired: 2 in, 2 out]
              }
            }
          }
          frame "Comp_Res_Meas" {
            w328 = 2  # time
            w332 = 1  # date
            w319 = "F" ("f")
            w320 = "P"
            w339 = 13  # p_f
            # "4"
            # "3"
            # "2"
            # "1"
            # "1. If the required value is greater than the open resistance value.\n2. If the measured value is greater than the required res. value.\n3. If 1 and 2 pass, then indicate PASS.\n4. If 1 is true, use result of 3.  Use this for testing case of open resistance."
            # "Make sure we are within certain percentage."
            n139 = Unbundle By Name(w349) -> ("meas_res_str"=w348:string, "sw_pins"=w347:string[][], "port_row"=w329:i32, "Table Control"=w340:T3)
            n140 = Index Array(array=w347, index (row) #1=w329, index (col) #1=2 ("disabled index (col)"), index (row) #2=w329, index (col) #2=4 ("index (col)")) -> (element #1=w345:string, element #2=w343:string)
            n141 = Get Date/Time String(want seconds? (F)=TRUE) -> (date string=w330:string, time string=w327:string)  [unwired: 2 in]
            n142 = Fract/Exp String To Number(string=w348) -> (number=w323:dbl)  [unwired: 3 in, 1 out]
            n143 = Fract/Exp String To Number(string=w345) -> (number=w322:dbl)  [unwired: 3 in, 1 out]
            n144 = Fract/Exp String To Number(string=w343) -> (number=w342:dbl)  [unwired: 3 in, 1 out]
            n145 = Divide(x=w342, y=100.0) -> (x/y=w337:dbl)
            n146 = Greater Or Equal?(x=w322, y="open_res") -> (x >= y?=w314:bool)
            n147 = Multiply(x=w322, y=w337) -> (x*y=w336:dbl)
            n148 = Add(x=w322, y=w336) -> (x+y=w335:dbl)
            n149 = Subtract(x=w322, y=w336) -> (x-y=w334:dbl)
            n150 = Greater?(x=w323, y=w322) -> (0:w318:bool)
            n151 = In Range and Coerce(upper limit=w335, x=w323, lower limit=w334) -> (In Range?=w338:bool)  [unwired: 1 out]
            n152 = And(x=w314, y=w318) -> (x .and. y?=w321:bool)
            n153 = Select(t=w320, s=w321, f=w319) -> (s? t:f=w317:string)
            n154 = Select(t=w320, s=w338, f=w319) -> (s? t:f=w316:string)
            n155 = Select(t=w317, s=w314, f=w316) -> (s? t:f=w315:string)
            n156 = Replace Array Subset(array=w340, new element #1=w315, index (row) #1=w329, index (col) #1=w339, new element #2=w330, index (row) #2=w329, index (col) #2=w332, new element #3=w327, index (row) #3=w329, index (col) #3=w328) -> (w333:T3)
            n157 = Bundle By Name(cluster=w349, "main_states"=states."Disp_Meas", "Table Control"=w333) -> (w325:T6)
            n158 = local write "Table Control"(w333) -> ()
            n159 = Enqueue Element(queue=w352, element=w325) -> (error out=w350:errorcluster)  [unwired: 2 in, 2 out]
          }
          frame "Disp_Meas" {
            # "Update the Table Control on the\nfront panel."
            n160 = Unbundle By Name(w354) -> ("Table Control"=w355:T3)
            n161 = Bundle By Name(cluster=w354, "main_states"=states."Open_ports") -> (w353:T6)
            n162 = local write "Table Control"(w355) -> ()
            n163 = Enqueue Element(queue=w359, element=w353) -> (error out=w357:errorcluster)  [unwired: 2 in, 2 out]
          }
          frame "Incr_File_Name" {
            # "Increment the file name if we are cycling\nthe resistance test."
            n164 = local read "file_name_path"() -> (w371:path)
            n165 = local read "cyc_cntr_ind"() -> (w373:u32)
            n166 = Strip Path(path=w371) -> (stripped path=w360:path, name=w369:string)
            n167 = Number To Decimal String(number=w373) -> (decimal integer string=w367:string)  [unwired: 1 in]
            n168 = Match Pattern(string=w369, regular expression="[.]") -> (before substring=w361:string)  [unwired: 1 in, 3 out]
            n169 = Concatenate Strings(w361, "_" ("string"), w367, ".csv" ("string")) -> (w366:string)
            n170 = Build Path(base path=w360, name or relative path=w366) -> (appended path=w372:path)
            n171 = Open/Create/Replace File(file path (use dialog)=w372, operation (0:open)=T7."open or create") -> (refnum out=w364:refnum<file>)  [unwired: 4 in, 2 out]
            n172 = Bundle By Name(cluster=w374, "main_states"=states."Store_Res_Meas", "file_name_incr"=w364) -> (w363:T6)
            n173 = Enqueue Element(queue=w378, element=w363) -> (error out=w376:errorcluster)  [unwired: 2 in, 2 out]
          }
          frame "Store_Res_Meas" {
            w381 = "%s" ("format string")
            w380 = "," ("delimiter (Tab)")
            # "1.  If we didn't create a file or increment a file, then\n     use the file that is in the path field."
            # "1"
            # "Save information from table\ncontrol into a spreadsheet."
            n174 = Unbundle By Name(w398) -> ("file_name_incr"=w397:refnum<file>, "file_name_ref"=w396:refnum<file>, "Table Control"=w385:T3)
            n175 = local read "cycle"() -> (w395:bool)
            n176 = property on="Table Control" class="Tbl (strict)"() -> ("Column Headers[]"=w384:string[])  [unwired: 2 in, 2 out]
            n177 = local read "file_name_path"() -> (w389:path)
            n178 = Select(t=states."Fin_Cyc_Qry" ("main_states"), s=w395, f=states."Disable_SMU") -> (s? t:f=w392:T1)
            n179 = Select(t=w397, s=w395, f=w396) -> (s? t:f=w387:refnum<file>)
            n180 = Get File Size(file=w389) -> (refnum out=w388:refnum<file>)  [unwired: 1 in, 2 out]
            n181 = Equal?(x=w387, y=refnum<file> refnum) -> (x = y?=w390:bool)
            n182 = Select(t=w388, s=w390, f=w387) -> (s? t:f=w386:refnum<file>)
            n183 = Array To Spreadsheet String(delimiter (Tab)=w380, array=w385, 3:w381) -> (spreadsheet string=w399:string)
            n184 = Array To Spreadsheet String(delimiter (Tab)=w380, array=w384, 3:w381) -> (spreadsheet string=w382:string)
            n185 = Concatenate Strings(w382, w399) -> (w383:string)
            n186 = Bundle By Name(cluster=w398, "main_states"=w392) -> (w379:T6)
            n187 = Write to Text File(file (use dialog)=w386, text=w383) -> ()  [unwired: 2 in, 3 out]
            n188 = Enqueue Element(queue=w402, element=w379) -> (error out=w400:errorcluster)  [unwired: 2 in, 2 out]
          }
          frame "Finish_Test_Qry" {
            # "2"
            # "1"
            # "1.  Check to see if we are finished with the test.\n2.  Reset to row 0 if finished."
            n189 = Unbundle By Name(w417) -> ("num_of_meas"=w413:i32, "port_row"=w416:i32, "cyc_cntr_ind"=w409:u32, "Table Control"=w407:T3)
            n190 = Decrement(x=w413) -> (x-1=w412:i32)
            n191 = Increment(x=w409) -> (x+1=w411:u32)
            n192 = Equal?(x=w412, y=w416) -> (x = y?=w408:bool)
            n193 = Select(t=states."Cycling_Qry" ("main_states"), s=w408, f=states."Go_to_nxt_meas" ("main_states")) -> (s? t:f=w404:T1)
            n194 = Select(t=0, s=w408, f=w416) -> (s? t:f=w414:i32)
            n195 = Select(t=w411, s=w408, f=w409) -> (s? t:f=w410:u32)
            n196 = Select(t=w407, s=w408, f=w407) -> (s? t:f=w406:T3)
            n197 = Bundle By Name(cluster=w417, "main_states"=w404, "port_row"=w414, "cyc_cntr_ind"=w410, "Table Control"=w406) -> (w403:T6)
            n198 = local write "cyc_cntr_ind"(w410) -> ()
            n199 = Enqueue Element(queue=w421, element=w403) -> (error out=w418:errorcluster)  [unwired: 2 in, 2 out]
          }
          frame "Go_to_nxt_meas" {
            # "1"
            # "1. Increment port row to go to the next switching set."
            n200 = Unbundle By Name(w427) -> ("port_row"=w426:i32, "Table Control"=w424:T3)
            n201 = Increment(x=w426) -> (x+1=w425:i32)
            n202 = Bundle By Name(cluster=w427, "main_states"=states."Close_ports", "port_row"=w425, "Table Control"=w424) -> (w422:T6)
            n203 = Enqueue Element(queue=w430, element=w422) -> (error out=w428:errorcluster)  [unwired: 2 in, 2 out]
          }
          frame "Search cPCI Pin" {
            w433 = 3  # net_name
            w436 = 6  # net_name_2
            w437 = 5  # net_name_1
            w449 = 1  # cPCI_pin
            # "1"
            # "1.  Map the first or second pin reference designation with\nthe mapping file.  This will tell us the index of\nall the other information about this cpci pin.\n2.  Update the table control."
            n204 = Unbundle By Name(w452) -> ("first_port_arry"=w446:string[], "second_port_arry"=w445:string[], "port_row"=w440:i32, "map_table"=w443:string[][], "first_port_flg"=w438:bool, "Table Control"=w441:T3)
            n205 = Select(t=w446, s=w438, f=w445) -> (s? t:f=w444:string[])
            n206 = Select(t=w437, s=w438, f=w436) -> (s? t:f=w435:i32)
            n207 = Index Array(array=w444, index=w440) -> (element=w447:string)
            n208 = Index Array(array=w443, index (col)=w449) -> (element=w448:string[])  [unwired: 1 in]
            n209 = Search 1D Array(1D array=w448, element=w447) -> (index of element=w442:i32)  [unwired: 1 in]
            n210 = Index Array(array=w443, index (row)=w442, index (col)=w433) -> (element=w439:string)
            n211 = Replace Array Subset(array=w441, new element=w439, index (row)=w440, index (col)=w435) -> (w434:T3)
            n212 = Bundle By Name(cluster=w452, "main_states"=states."Select Adj Col Cnt", "port_indx_row"=w442, "Table Control"=w434) -> (w432:T6)
            n213 = local write "Table Control"(w434) -> ()
            n214 = Enqueue Element(queue=w453, element=w432) -> (error out=w450:errorcluster)  [unwired: 2 in, 2 out]
          }
          frame "Select Adj Col Cnt" {
            w456 = 0  # switch_col
            w474 = 7  # cpci_map
            w466 = 3  # J4_col
            w465 = 1  # J3_col
            # "1.  Determine whether we will use the J3 or J4\n     column of the 3732 card if we are using the 156 pins BOB.\n2.  Determine whether to use the BOB or cPCI mapping\n     column.\n3.  Port 1 will use row 3 and port 2 will use row 4.\n4.  Bank will always be 1.\n5.  This is the column that the switch will use for either\n     port 1 or port 2 of the resistor measurment.\n6.  Choose between the 156 or 78 pins BOB.  For the 78 pins BOB,\n     we just need to look at column 0 of the mapping file.  All the\n     switching columns are unique.  Don't need to use point 8 \n     below.\n7.  If the column is less than 10, add 0 in front of it.\n8.  If the pin count is above 56, use the J4 col for the 78 pins BOB."
            # "8"
            # "7"
            # "6"
            # "2"
            # "5"
            # "4"
            # "3"
            # "1"
            n215 = Unbundle By Name(w495) -> ("first_port_arry"=w486:string[], "second_port_arry"=w485:string[], "port_row"=w477:i32, "map_table"=w492:string[][], "port_indx_row"=w491:i32, "first_port_flg"=w487:bool)
            n216 = local read "bob_156"() -> (w472:bool)
            n217 = local read "bob_78"() -> (w475:bool)
            n218 = Select(t=w486, s=w487, f=w485) -> (s? t:f=w480:string[])
            n219 = Select(t="3" ("bank_number"), s=w487, f="4") -> (s? t:f=w479:string)
            n220 = Index Array(array=w480, index=w477) -> (element=w470:string)
            n221 = String Subset(string=w470, length (rest)=2 ("length (rest)")) -> (substring=w484:string)  [unwired: 1 in]
            n222 = Decimal String To Number(string=w470) -> (number=w469:i32)  [unwired: 2 in, 1 out]
            n223 = Greater?(x=w469, y=56) -> (0:w467:bool)
            n224 = Match True/False String(2:"J4" ("false string"), 3:"J3" ("true string"), 4:w484) -> (0:w473:bool)  [unwired: 1 out]
            n225 = Select(t=w465, s=w473, f=w466) -> (s? t:f=w471:i32)
            n226 = Select(t=w466, s=w467, f=w465) -> ()  [unwired: 1 out]
            n227 = Or(x=w472, y=w475) -> (x .or. y?=w476:bool)
            n228 = Select(t=w471, s=w472, f=w456) -> (s? t:f=w464:i32)
            n229 = Select(t=w464, s=w476, f=w474) -> (s? t:f=w478:i32)
            n230 = Index Array(array=w492, index (row)=w491, index (col)=w478) -> (element=w458:string)
            n231 = String Length(string=w458) -> (length=w463:i32)
            n232 = Equal?(x=w463, y=1) -> (x = y?=w460:bool)
            n233 = Concatenate Strings("0" ("string"), w458) -> (w459:string)
            n234 = Select(t=w459, s=w460, f=w458) -> (s? t:f=w457:string)
            n235 = Bundle By Name(cluster=w495, "main_states"=states."Sel Slot Number", "adj_col_cnt"=w457, "bank_number"="1", "row_number"=w479) -> (w454:T6)
            n236 = Enqueue Element(queue=w496, element=w454) -> (error out=w493:errorcluster)  [unwired: 2 in, 2 out]
          }
          frame "Sel Slot Number" {
            w505 = 11  # slot_number
            # "2"
            # "1"
            # "1.  Select the slot number according to the\npin count from the nets_updated mapping file if\nusing the cPCI fixture.\n2.  If using the BOB, we get the slot number from\nthe ports list."
            n237 = Unbundle By Name(w538) -> ("map_table"=w535:string[][], "port_indx_row"=w533:i32, "first_port_flg"=w510:bool, "sw_pins"=w506:string[][], "port_row"=w504:i32)
            n238 = local read "bob_156"() -> (w501:bool)
            n239 = local read "bob_78"() -> (w500:bool)
            n240 = Select(t=states."Build 1st Port SBRCC Code" ("main_states"), s=w510, f=states."Build 2nd Port SBRCC Code") -> (s? t:f=w498:T1)
            n241 = Or(x=w501, y=w500) -> (x .or. y?=w499:bool)
            n242 = Index Array(array=w535, index (row)=w533, index (col)=0 ("disabled index (col)")) -> (element=w532:string)
            n243 = Index Array(array=w506, index (row)=w504, index (col)=w505) -> (element=w503:string)
            n244 = Decimal String To Number(string=w532) -> (number=w516:i32)  [unwired: 2 in, 1 out]
            n245 = Less?(x=w516, y=113) -> (x < y?=w530:bool)
            n246 = Less?(x=w516, y=225) -> (x < y?=w527:bool)
            n247 = Less?(x=w516, y=337) -> (x < y?=w524:bool)
            n248 = Less?(x=w516, y=449) -> (x < y?=w521:bool)
            n249 = Less?(x=w516, y=561) -> (x < y?=w518:bool)
            n250 = Select(t="5" ("bank_number"), s=w518, f="6") -> (s? t:f=w511:string)
            n251 = Select(t="4" ("bank_number"), s=w521, f=w511) -> (s? t:f=w512:string)
            n252 = Select(t="3" ("bank_number"), s=w524, f=w512) -> (s? t:f=w513:string)
            n253 = Select(t="2" ("bank_number"), s=w527, f=w513) -> (s? t:f=w514:string)
            n254 = Select(t="1" ("bank_number"), s=w530, f=w514) -> (s? t:f=w507:string)
            n255 = Select(t=w503, s=w499, f=w507) -> (s? t:f=w502:string)
            n256 = Bundle By Name(cluster=w538, "main_states"=w498, "slot_number"=w502) -> (w497:T6)
            n257 = Enqueue Element(queue=w539, element=w497) -> (error out=w536:errorcluster)  [unwired: 2 in, 2 out]
          }
          frame "Build 1st Port SBRCC Code" {
            w544 = 7  # col_1_switch
            # "2"
            # "1"
            # "1.  Combine all the switching information\nfor column 1.\n2.  Update the table control."
            n258 = Unbundle By Name(w555) -> ("first_port_col"=w552:string[], "port_row"=w545:i32, "slot_number"=w551:string, "bank_number"=w550:string, "row_number"=w549:string, "adj_col_cnt"=w548:string, "Table Control"=w546:T3)
            n259 = Concatenate Strings(w551, w550, w549, w548) -> (w543:string)
            n260 = Replace Array Subset(array=w552, new element=w543, index=w545) -> (w547:string[])
            n261 = Replace Array Subset(array=w546, new element=w543, index (row)=w545, index (col)=w544) -> (w542:T3)
            n262 = Bundle By Name(cluster=w555, "main_states"=states."Clr_1st_port_flg", "first_port_col"=w547, "Table Control"=w542) -> (w541:T6)
            n263 = local write "Table Control"(w542) -> ()
            n264 = Enqueue Element(queue=w556, element=w541) -> (error out=w553:errorcluster)  [unwired: 2 in, 2 out]
          }
          frame "Build 2nd Port SBRCC Code" {
            w560 = 8  # col_2_switch
            # "2"
            # "1"
            # "1.  Combine all the switching information\nfor column 2.\n2.  Update the table control."
            n265 = Unbundle By Name(w572) -> ("second_port_col"=w569:string[], "port_row"=w561:i32, "slot_number"=w568:string, "bank_number"=w567:string, "row_number"=w566:string, "adj_col_cnt"=w565:string, "Table Control"=w563:T3)
            n266 = Concatenate Strings(w568, w567, w566, w565) -> (w559:string)
            n267 = Replace Array Subset(array=w569, new element=w559, index=w561) -> (w564:string[])
            n268 = Replace Array Subset(array=w563, new element=w559, index (row)=w561, index (col)=w560) -> (w562:T3)
            n269 = Bundle By Name(cluster=w572, "main_states"=states."Clr_2nd_port_flg", "second_port_col"=w564, "Table Control"=w562) -> (w557:T6)
            n270 = local write "Table Control"(w562) -> ()
            n271 = Enqueue Element(queue=w573, element=w557) -> (error out=w570:errorcluster)  [unwired: 2 in, 2 out]
          }
          frame "Set AB4 Code" {
            w577 = 9  # ab_switch
            # "4"
            # "3"
            # "1"
            # "1.  Only need to concatenate the slot number.\n3.  Update the table control.\n4.  Move to the next row."
            n272 = Unbundle By Name(w588) -> ("ab_code"=w585:string[], "port_row"=w578:i32, "slot_number"=w584:string, "Table Control"=w580:T3)
            n273 = Increment(x=w578) -> (x+1=w581:i32)
            n274 = Concatenate Strings(w584, "0914" ("string")) -> (w576:string)
            n275 = Replace Array Subset(array=w585, new element=w576, index=w578) -> (w583:string[])
            n276 = Replace Array Subset(array=w580, new element=w576, index (row)=w578, index (col)=w577) -> (w579:T3)
            n277 = Bundle By Name(cluster=w588, "main_states"=states."Finish_port_match_qry", "ab_code"=w583, "port_row"=w581, "Table Control"=w579) -> (w574:T6)
            n278 = local write "Table Control"(w579) -> ()
            n279 = Enqueue Element(queue=w589, element=w574) -> (error out=w586:errorcluster)  [unwired: 2 in, 2 out]
          }
          frame "Pop Cons Data" {
            # "Data from the producer loop."
            n280 = Unbundle By Name(w593) -> ("map_table"=w597:string[][], "sw_pins"=w595:string[][], "num_of_meas"=w594:i32, "file_name_ref"=w592:refnum<file>)
            n281 = Bundle By Name(cluster=w596, "main_states"=states."Idle", "map_table"=w597, "sw_pins"=w595, "num_of_meas"=w594, "file_name_ref"=w592) -> (w591:T6)
            n282 = Enqueue Element(queue=w600, element=w591) -> (error out=w598:errorcluster)  [unwired: 2 in, 2 out]
          }
          frame "Cycling_Qry" {
            w611 = FALSE ("y")
            w609 = TRUE ("y")
            # "4"
            # "1.  If cycling is true and save is true.\n2.  If cycling is true and save is false.\n3.  If cycling is false and save is true.\n4.  If cycling is false and save is false."
            # "3"
            # "2"
            # "1"
            # "Determine what to do after\nwe finish our testing set.  Not\ncycling set."
            n283 = local read "cycle"() -> (w612:bool)
            n284 = local read "save_file_qry"() -> (w610:bool)
            n285 = Equal?(x=w612, y=w609) -> (x = y?=w617:bool)
            n286 = Equal?(x=w610, y=w611) -> (x = y?=w616:bool)
            n287 = Equal?(x=w612, y=w611) -> (x = y?=w608:bool)
            n288 = Equal?(x=w610, y=w609) -> (x = y?=w607:bool)
            n289 = And(x=w612, y=w610) -> (x .and. y?=w618:bool)
            n290 = And(x=w617, y=w616) -> (x .and. y?=w614:bool)
            n291 = And(x=w608, y=w607) -> (x .and. y?=w606:bool)
            n292 = Select(t=states."Store_Res_Meas" ("f"), s=w606, f=states."Disable_SMU") -> (s? t:f=w603:T1)
            n293 = Select(t=states."Fin_Cyc_Qry" ("f"), s=w614, f=w603) -> (s? t:f=w604:T1)
            n294 = Select(t=states."Incr_File_Name" ("main_states"), s=w618, f=w604) -> (s? t:f=w620:T1)
            n295 = Bundle By Name(cluster=w619, "main_states"=w620) -> (w601:T6)
            n296 = Enqueue Element(queue=w623, element=w601) -> (error out=w621:errorcluster)  [unwired: 2 in, 2 out]
          }
          frame "Fin_Cyc_Qry" {
            # "Determine if we are finished\nwith the cycling routine."
            n297 = Unbundle By Name(w625) -> ("cyc_cntr"=w629:u32)
            n298 = local read "num_of_cycles"() -> (w628:u32)
            n299 = Decrement(x=w628) -> (x-1=w627:u32)
            n300 = Equal?(x=w629, y=w627) -> (x = y?=w626:bool)
            n301 = Select(t=states."Disable_SMU" ("main_states"), s=w626, f=states."Test_Cancel_Qry") -> (s? t:f=w630:T1)
            n302 = Bundle By Name(cluster=w625, "main_states"=w630) -> (w624:T6)
            n303 = Enqueue Element(queue=w635, element=w624) -> (error out=w633:errorcluster)  [unwired: 2 in, 2 out]
          }
          frame "Clr_Cyc_Cntr" {
            w636 = FALSE ("strt_meas")
            # "Clear cycling counter and go to idle."
            n304 = Bundle By Name(cluster=w640, "main_states"=states."Idle", "cyc_cntr"=u32 0) -> (w637:T6)
            n305 = local write "strt_meas"(w636) -> ()
            n306 = local write "cycle"(w636) -> ()
            n307 = Enqueue Element(queue=w643, element=w637) -> (error out=w641:errorcluster)  [unwired: 2 in, 2 out]
          }
          frame "Test_Cancel_Qry" {
            # "Determine if the test is being cancel."
            n308 = local read "strt_meas"() -> (w648:bool)
            n309 = Select(t=states."Clr_Table_Cols" ("main_states"), s=w648, f=states."Disable_SMU") -> (s? t:f=w645:T1)
            n310 = Bundle By Name(cluster=w649, "main_states"=w645) -> (w644:T6)
            n311 = Enqueue Element(queue=w652, element=w644) -> (error out=w650:errorcluster)  [unwired: 2 in, 2 out]
          }
          frame "Incr_cyc_cntr" {
            w654 = 2  # time
            w655 = 1  # date
            w656 = 13  # p_f
            w653 = string[] ["", "", "", "", "", "", "", "", "", "", "", "", "", "", "", "", "", "", "", "", "", "", "", "", "", "", "", "", "", "", "", "", "", "", "", "", "", "", "", "", "", "", "", "", "", "", "", "", "", "", "", "", "", "", "", "", "", "", "", "", "", "", "", "", "", "", "", "", "", "", "", "", "", "", "", "", "", "", "", "", "", "", "", "", "", "", "", "", "", "", "", "", "", "", "", "", "", "", "", "", "", "", "", "", "", "", "", "", "", "", "", "", "", "", "", "", "", "", "", "", "", "", "", "", "", "", "", "", "", "", "", "", "", "", "", "", "", "", "", "", "", "", "", "", "", "", "", "", "", "", "", "", "", "", "", "", "", "", "", "", "", "", "", "", "", "", "", "", "", "", "", "", "", "", "", "", "", "", "", "", "", "", "", "", "", "", "", "", "", "", "", "", "", "", "", "", "", "", "", "", "", "", "", "", "", "", "", "", "", "", "", "", "", "", "", "", "", "", "", "", "", "", "", "", "", "", "", "", "", "", "", "", "", "", "", "", "", "", "", "", "", "", "", "", "", "", "", "", "", "", "", "", "", "", "", "", "", "", "", "", "", "", "", "", "", "", "", "", "", "", "", "", "", "", "", "", "", "", "", "", "", "", "", "", "", "", "", "", "", "", "", "", "", "", "", "", "", "", "", "", "", "", "", "", "", "", "", "", "", "", "", "", "", "", "", "", "", "", "", "", "", "", "", "", "", "", "", "", "", "", "", "", "", "", "", "", "", "", "", "", "", "", "", "", "", "", "", "", "", "", "", "", "", "", "", "", "", "", "", "", "", "", "", "", "", "", "", "", "", "", "", "", "", "", "", "", "", "", "", "", "", "", "", "", "", "", "", "", "", "", "", "", "", "", "", "", "", "", "", "", "", "", "", "", "", "", "", "", "", "", "", "", "", "", "", "", "", "", "", "", "", "", "", "", "", "", "", "", "", "", "", "", "", "", "", "", "", "", "", "", "", "", "", "", "", "", "", "", "", "", "", "", "", "", "", "", "", "", "", "", "", "", "", "", "", "", "", "", "", "", "", "", "", "", "", "", "", "", "", "", "", "", "", "", "", "", "", "", "", "", "", "", "", "", "", "", "", "", "", "", "", "", "", "", "", "", "", "", "", "", "", "", "", "", "", "", "", "", "", "", "", "", "", "", "", "", "", "", "", "", "", "", "", "", "", "", "", "", "", "", "", "", "", "", "", "", "", "", "", "", "", "", "", "", "", "", "", "", "", "", "", "", "", "", "", "", "", "", "", "", "", "", "", "", "", "", "", "", "", "", "", "", "", "", "", "", "", "", "", "", "", "", "", "", "", "", "", "", "", " "] ("new element/subarray")
            w657 = 11  # meas_val
            # "2"
            # "1"
            # "1.  Increment cycle counter and\n     start test again.\n2.  Clear the measured value column\n     and the p/f result column."
            n312 = Unbundle By Name(w664) -> ("cyc_cntr"=w663:u32, "Table Control"=w659:T3)
            n313 = Increment(x=w663) -> (x+1=w660:u32)
            n314 = Replace Array Subset(array=w659, new element #1=w653, index (col) #1=w657, new element #2=w653, index (col) #2=w656, new element #3=w653, index (col) #3=w655, new element #4=w653, index (col) #4=w654) -> (w658:T3)  [unwired: 4 in]
            n315 = Bundle By Name(cluster=w664, "cyc_cntr"=w660, "main_states"=states."Close_ports", "Table Control"=w658) -> (w661:T6)
            n316 = Enqueue Element(queue=w667, element=w661) -> (error out=w665:errorcluster)  [unwired: 2 in, 2 out]
          }
          frame "Clr_Table_Cols" {
            # "Increment cycle counter and\nstart test again."
            n317 = Unbundle By Name(w672) -> ("Table Control"=w669:T3, "cyc_cntr"=→"cyc_cntr_ind":u32)
            n318 = Bundle By Name(cluster=w672, "main_states"=states."Incr_cyc_cntr", "Table Control"=w669) -> (w670:T6)
            n319 = Enqueue Element(queue=w675, element=w670) -> (error out=w673:errorcluster)  [unwired: 2 in, 2 out]
          }
          frame "clr_queue" {
            n320 = Flush Queue(queue=w681) -> (queue out=w676:refnum<queue>)  [unwired: 1 in, 2 out]
            n321 = Bundle By Name(cluster=w682, "main_states"=states."Idle") -> (w678:T6)
            n322 = Enqueue Element(queue=w676, element=w678) -> (error out=w679:errorcluster)  [unwired: 2 in, 2 out]
          }
        }
      }
      frame Error {
        # "Return true in any case that should stop the loop."
      }
    }
  }
  n323 = while {
    shift-right: [w695] -> w22
    shift-left: w23 -> [w697]
    tunnel: w21 -> [w698]
    tunnel: w8 -> [w692]
    tunnel: [w691] -> w18
    shift-right: [w689] -> w17
    shift-left: w7 -> [w690]
    shift-right: [w688] -> _
    shift-left: w2 -> [w693]
    stop <- w687 stop-if-true
    # "Generate user events."
    # "This loop is the producer loop."
    n324 = event shown="[3] \"strt_meas\": Value Change" {
      selector: w692 -> [_ _ _ _ _ _ _ _ _ _ _ _ _ _ _ _ _ _ _ _ _ _]
      dyn-events: [_ _ _ _ _ _ _ _ _ _ _ _ _ _ _ _ _ _ _ _ _ _] -> w691
      timeout: _ -> [_ _ _ _ _ _ _ _ _ _ _ _ _ _ _ _ _ _ _ _ _ _]
      tunnel: w698 -> [_ w713 w747 w759 _ _ _ w806 w818 _ _ _ _ _ _ _ _ _ _ _ _ _]
      tunnel: w697 -> [_ w715 w750 w758 w777 w783 w796 _ _ w825 w833 w841 w849 w853 w860 w870 w874 w885 w891 w895 w942 w949]
      tunnel: [w700 w714 w749 w757 w777 w783 w796 w804 w816 w824 w832 w840 w848 w853 w860 w870 w874 w885 w891 w894 w942 w949] -> w695
      tunnel: ["stop" FALSE ("stop") FALSE ("stop") FALSE ("stop") FALSE ("stop") FALSE ("stop") FALSE ("stop") FALSE ("stop") FALSE ("stop") FALSE ("stop") FALSE ("stop") FALSE ("stop") FALSE ("stop") FALSE ("stop") FALSE ("stop") FALSE ("stop") FALSE ("stop") FALSE ("stop") FALSE ("stop") FALSE ("stop") FALSE ("stop") FALSE ("stop")] -> w696
      tunnel: w693 -> [w701 w706 w748 w755 w774 w780 w797 w805 w817 w823 w831 w839 w847 w855 w862 w872 w876 w887 w893 w899 w946 w953]
      tunnel: w690 -> [w703 w707 w744 w754 w778 w784 w798 w808 w820 w826 w834 w842 w850 w854 w861 w871 w875 w886 w892 w898 w945 w952]
      tunnel: [w703 w709 w745 w754 w778 w784 w798 w808 w820 w826 w834 w842 w850 w854 w861 w871 w875 w886 w892 w898 w945 w952] -> w689
      tunnel: [w701 w705 w741 w753 w773 w779 w794 w802 w812 w823 w831 w839 w847 w855 w862 w872 w876 w887 w893 w899 w946 w953] -> w688
      event "stop": Value Change {
        n325 = event-data() -> ()  [unwired: 1 in, 1 out]
        n326 = Unbundle By Name(w701) -> ("sw_visa_res_out"=w702:refnum<visa-resource-name>, "smu_visa_res_out"=w699:refnum<visa-resource-name>)
        n327 = call <instrlib>:"ke37xx Close.vi"("VISA resource name"=w702) -> ("error out"=w700:errorcluster)  [unwired: 14 in]
        n328 = call <instrlib>:"Close.vi"("VISA resource name"=w699) -> ()  [unwired: 10 in, 1 out]
      }
      event "create_file": Value Change {
        n329 = event-data() -> ()  [unwired: 1 in, 1 out]
        n330 = local read "file_name_path"() -> (w711:path)
        n331 = File/Directory Info(path=w711, error in=w707) -> (path out=w708:path, directory=w710:bool)  [unwired: 5 out]
        n332 = case shown="False" w710 {
          tunnel: T7."replace or create" ("operation (0:open)") -> [w729 w740]
          tunnel: w706 -> [w727 w737]
          tunnel: [w726 w736] -> w705
          tunnel: states."Pop Cons Data" ("main_states") -> [w725 w735]
          tunnel: w707 -> [w721 w733]
          tunnel: [w720 w732] -> w709
          tunnel: w708 -> [w719 w731]
          frame False {
            # "If the directory does not exist, create it and the file."
            n333 = Strip Path(path=w719) -> (stripped path=w723:path, name=w718:string)
            n334 = Create Folder(path (use dialog)=w723, error in=w721) -> (created path=w722:path)  [unwired: 1 in, 2 out]
            n335 = Build Path(base path=w722, name or relative path=w718) -> (appended path=w728:path)
            n336 = Open/Create/Replace File(file path (use dialog)=w728, operation (0:open)=w729) -> (refnum out=w724:refnum<file>, error out=w720:errorcluster)  [unwired: 4 in, 1 out]
            n337 = Bundle By Name(cluster=w727, "file_name_ref"=w724, "main_states"=w725) -> (w726:T6)
          }
          frame True {
            # "If the directory exists, create file only."
            n338 = Strip Path(path=w731) -> (stripped path=w739:path, name=w730:string)
            n339 = Build Path(base path=w739, name or relative path=w730) -> (appended path=w738:path)
            n340 = Open/Create/Replace File(file path (use dialog)=w738, error in=w733, operation (0:open)=w740) -> (refnum out=w734:refnum<file>, error out=w732:errorcluster)  [unwired: 3 in, 1 out]
            n341 = Bundle By Name(cluster=w737, "file_name_ref"=w734, "main_states"=w735) -> (w736:T6)
          }
        }
        n342 = Enqueue Element(queue=w713, element=w705, error in (no error)=w715) -> (error out=w714:errorcluster)  [unwired: 1 in, 2 out]
      }
      event "file_name_path": Value Change {
        # "If the user chooses a file, pass it to the\nconsumer loop for saving data later."
        n343 = event-data() -> ()  [unwired: 1 in, 1 out]
        n344 = local read "file_name_path"() -> (w743:path)
        n345 = Get File Size(file=w743, error in=w744) -> (refnum out=w742:refnum<file>, 0:w745:errorcluster)  [unwired: 1 out]
        n346 = Bundle By Name(cluster=w748, "file_name_ref"=w742, "main_states"=states."Pop Cons Data") -> (w741:T6)
        n347 = Enqueue Element(queue=w747, element=w741, error in (no error)=w750) -> (error out=w749:errorcluster)  [unwired: 1 in, 2 out]
      }
      event "strt_meas": Value Change {
        n348 = event-data() -> ("NewVal"=w752:bool)  [unwired: 1 in]
        n349 = case shown="True" w752 {
          tunnel: w759 -> [w766 w772]
          tunnel: w758 -> [w765 w771]
          tunnel: [w764 w770] -> w757
          tunnel: w755 -> [w763 w769]
          tunnel: [w761 w767] -> w753
          frame True {
            n350 = property on="Table Control" class="Tbl (strict)"("Value"=string[][] array600x14[8400 elements] ("cpci_table")) -> ()  [unwired: 2 in, 2 out]
            n351 = Bundle By Name(cluster=w763, "main_states"=states."Set_SMU_Current") -> (w761:T6)
            n352 = Enqueue Element(queue=w766, element=w761, error in (no error)=w765) -> (error out=w764:errorcluster)  [unwired: 1 in, 2 out]
          }
          frame False {
            n353 = Bundle By Name(cluster=w769, "main_states"=states."clr_queue") -> (w767:T6)
            n354 = Enqueue Element(queue=w772, element=w767, error in (no error)=w771) -> (error out=w770:errorcluster)  [unwired: 1 in, 2 out]
          }
        }
      }
      event User Event {
        # "grab the visa resource after\ninitialization"
        n355 = event-data() -> ("sw_visa_res_out"=w775:refnum<visa-resource-name>)  [unwired: 1 in, 2 out]
        n356 = Bundle By Name(cluster=w774, "sw_visa_res_out"=w775) -> (w773:T6)
      }
      event User Event {
        # "grab the visa resource after\ninitialization"
        n357 = event-data() -> ("smu_visa_res_out"=w781:refnum<visa-resource-name>)  [unwired: 1 in, 2 out]
        n358 = Bundle By Name(cluster=w780, "smu_visa_res_out"=w781) -> (w779:T6)
      }
      event User Event {
        n359 = event-data() -> ("first_port_arry"=w793:string[], "second_port_arry"=w792:string[], "first_port_col"=w791:string[], "second_port_col"=w790:string[], "num_of_meas"=w789:i32, "sw_visa_res_out"=w788:refnum<visa-resource-name>, "map_table"=w787:string[][], "sw_pins"=w786:string[][], "smu_visa_res_out"=w785:refnum<visa-resource-name>)  [unwired: 1 in]
        n360 = Bundle By Name(cluster=w797, "first_port_arry"=w793, "second_port_arry"=w792, "first_port_col"=w791, "second_port_col"=w790, "num_of_meas"=w789, "sw_visa_res_out"=w788, "map_table"=w787, "sw_pins"=w786, "smu_visa_res_out"=w785) -> (w794:T6)
      }
      event "map_path": Value Change {
        # "take the excel sheet and create a table of cpci pins and other\ninformation.  Also, take out the first row of column headers."
        n361 = event-data() -> ()  [unwired: 1 in, 3 out]
        n362 = local read "map_path"() -> (w801:path)
        n363 = call "Extract_csv_file.vi"("cpci_pins_path"=w801) -> ("text_table"=w799:string[][], "orig_text_table"=→"cpci_or_bob_table":string[][])  [unwired: 9 in]
        n364 = Bundle By Name(cluster=w805, "map_table"=w799, "main_states"=states."Pop Cons Data") -> (w802:T6)
        n365 = Enqueue Element(queue=w806, element=w802) -> (error out=w804:errorcluster)  [unwired: 2 in, 2 out]
      }
      event "ports_path": Value Change {
        # "take the excel sheet and create a table of the required switching\npins, ie, two pins to measure the resistor.  Also, take out the column headers row.  \nAlso, find out how many resistors we have to measure, ie rows."
        n366 = event-data() -> ()  [unwired: 1 in, 1 out]
        n367 = local read "ports_path"() -> (w810:path)
        n368 = call "Extract_csv_file.vi"("cpci_pins_path"=w810) -> ("text_table"=w809:string[][])  [unwired: 9 in, 1 out]
        "port_list" <- w809
        n369 = Index Array(array=w809, index (col)=0 ("disabled index (col)")) -> (element=w814:string[])  [unwired: 1 in]
        n370 = Array Size(array=w814) -> (size(s)=w813:i32)
        n371 = Bundle By Name(cluster=w817, "sw_pins"=w809, "num_of_meas"=w813, "main_states"=states."Pop Cons Data") -> (w812:T6)
        n372 = Enqueue Element(queue=w818, element=w812) -> (error out=w816:errorcluster)  [unwired: 2 in, 2 out]
      }
      event "close_port": Value Change {
        n373 = event-data() -> ()  [unwired: 1 in, 1 out]
        n374 = Unbundle By Name(w823) -> ("sw_visa_res_out"=w822:refnum<visa-resource-name>)
        n375 = call <instrlib>:"ke37xx Close Channels.vi"("VISA Resource Name"=w822, "Channel List"="cls_chnl_list", "error in (no error)"=w825) -> ("error out"=w824:errorcluster)  [unwired: 11 in, 1 out]
      }
      event "get_closed_list": Value Change {
        n376 = event-data() -> ()  [unwired: 1 in, 1 out]
        n377 = Unbundle By Name(w831) -> ("sw_visa_res_out"=w830:refnum<visa-resource-name>)
        n378 = call <instrlib>:"ke37xx Get Closed List.vi"("VISA Resource Name"=w830, "Channel List"="close_list", "error in (no error)"=w833) -> ("Closed List"=→"closed_list":string, "error out"=w832:errorcluster)  [unwired: 10 in, 1 out]
      }
      event "open_port": Value Change {
        n379 = event-data() -> ()  [unwired: 1 in, 1 out]
        n380 = Unbundle By Name(w839) -> ("sw_visa_res_out"=w838:refnum<visa-resource-name>)
        n381 = call <instrlib>:"ke37xx Open Channels.vi"("VISA Resource Name"=w838, "Channel List"="open_chnl_list", "Open All (False)"="open_all", "error in (no error)"=w841) -> ("error out"=w840:errorcluster)  [unwired: 10 in, 1 out]
      }
      event "config_bkplane": Value Change {
        n382 = event-data() -> ()  [unwired: 1 in, 1 out]
        n383 = Unbundle By Name(w847) -> ("sw_visa_res_out"=w846:refnum<visa-resource-name>)
        n384 = call <instrlib>:"ke37xx Configure Backplane.vi"("VISA Resource Name"=w846, "Channel List"="cls_chnl_list_bkpln", "Backplane Relays"="bkpl_relays", "error in (no error)"=w849) -> ("error out"=w848:errorcluster)  [unwired: 10 in, 1 out]
      }
      event "config_smu_funct": Value Change {
        n385 = event-data() -> ()  [unwired: 1 in, 2 out]
        n386 = disable-structure shown="Enabled" {
          disable-tunnel: w855 -> [w858 _]
          frame Enabled {
            n387 = Unbundle By Name(w858) -> ("smu_visa_res_out"=w857:refnum<visa-resource-name>)
            n388 = call "Config_Meas_Func.vi"("Function (0: Volts)"="config_smu_funct", "VISA resource name"=w857) -> ()  [unwired: 8 in, 2 out]
          }
          frame Disabled {
          }
        }
      }
      event "config_src": Value Change {
        n389 = event-data() -> ()  [unwired: 1 in, 2 out]
        n390 = disable-structure shown="Enabled" {
          disable-tunnel: w862 -> [w865 _]
          frame Enabled {
            n391 = Unbundle By Name(w865) -> ("smu_visa_res_out"=w863:refnum<visa-resource-name>)
            n392 = call <instrlib>:"Configure Source Function.vi"("Function (0: Volts)"="config_src", "VISA resource name"=w863) -> ()  [unwired: 8 in, 2 out]
          }
          frame Disabled {
          }
        }
      }
      event "read_smu_data": Value Change {
        n393 = event-data() -> ()  [unwired: 1 in, 1 out]
        n394 = Unbundle By Name(w872) -> ("smu_visa_res_out"=w868:refnum<visa-resource-name>)
        n395 = call <instrlib>:"Read (Single Point).vi"("VISA resource name"=w868) -> ("Data out"=w867:string)  [unwired: 12 in, 2 out]
        "smu_data" <- w867
        n396 = Fract/Exp String To Number(string=w867) -> (number=→"res_val":dbl)  [unwired: 3 in, 1 out]
      }
      event "src_mode", "src_level": Value Change {
        n397 = event-data() -> ()  [unwired: 1 in, 6 out]
        n398 = disable-structure shown="Enabled" {
          disable-tunnel: w876 -> [w880 _]
          frame Enabled {
            n399 = Unbundle By Name(w880) -> ("smu_visa_res_out"=w878:refnum<visa-resource-name>)
            n400 = call <instrlib>:"Configure Source Level.vi"("Source Level (1.0)"="src_level", "Function (0: Volts)"="src_mode", "VISA resource name"=w878) -> ()  [unwired: 7 in, 2 out]
          }
          frame Disabled {
          }
        }
      }
      event "src_lim": Value Change {
        n401 = event-data() -> ()  [unwired: 1 in, 1 out]
        n402 = Unbundle By Name(w887) -> ("smu_visa_res_out"=w883:refnum<visa-resource-name>)
        n403 = local read "src_mode"() -> (w881:u16)
        n404 = call <instrlib>:"Configure Source Limit Level.vi"("Source Limit (1.0)"="src_lim", "Function (0: Volts)"=w881, "VISA resource name"=w883) -> ()  [unwired: 7 in, 2 out]
      }
      event "enb_out": Value Change {
        n405 = event-data() -> ()  [unwired: 1 in, 6 out]
        n406 = Unbundle By Name(w893) -> ("smu_visa_res_out"=w889:refnum<visa-resource-name>)
        n407 = call <instrlib>:"Enable Output.vi"("Enable Output (T: Enable)"="enb_out", "VISA resource name"=w889) -> ()  [unwired: 8 in, 2 out]
      }
      event "config_meas_params": Value Change {
        n408 = event-data() -> ()  [unwired: 1 in, 1 out]
        n409 = Unbundle By Name(w899) -> ("smu_visa_res_out"=w896:refnum<visa-resource-name>)
        n410 = disable-structure shown="Enabled" {
          disable-tunnel: w896 -> [w913 w939]
          disable-tunnel: w895 -> [w910 _]
          disable-tunnel: [w907 w931] -> w894
          frame Disabled {
            n411 = disable-structure shown="Enabled" {
              disable-tunnel: w913 -> [w928 w930]
              disable-tunnel: [w924 w930] -> w904
              disable-tunnel: [w923 w929] -> w903
              disable-tunnel: w910 -> [w922 w929]
              frame Enabled {
                n412 = call <instrlib>:"Configure Measurement Range.vi"("Manual Range (1.0)"="Manual Range (1.0)", "error in (no error)"=w922, "Enable Auto Range (T:Enable)"="enb_auto_range", "Function (0: Volts)"="config_meas_type", "VISA resource name"=w928) -> ("error out"=w923:errorcluster, "VISA resource name out"=w924:refnum<visa-resource-name>)  [unwired: 5 in]
              }
              frame Disabled {
              }
            }
            n413 = local read "src_mode"() -> (w906:u16)
            n414 = local read "src_level"() -> (w909:dbl)
            n415 = call <instrlib>:"Configure Source Function.vi"("error in (no error)"=w903, "Function (0: Volts)"=w906, "VISA resource name"=w904) -> ("error out"=w902:errorcluster, "VISA resource name out"=w905:refnum<visa-resource-name>)  [unwired: 7 in]
            n416 = call <instrlib>:"Configure Source Level.vi"("error in (no error)"=w902, "Source Level (1.0)"=w909, "Function (0: Volts)"=w906, "VISA resource name"=w905) -> ("error out"=w911:errorcluster, "VISA resource name out"=w912:refnum<visa-resource-name>)  [unwired: 6 in]
            n417 = disable-structure shown="Disabled" {
              disable-tunnel: w912 -> [w919 w921]
              disable-tunnel: w911 -> [w918 w920]
              disable-tunnel: w906 -> [w916 _]
              disable-tunnel: [w915 w921] -> w901
              disable-tunnel: [w914 w920] -> w900
              frame Disabled {
                n418 = local read "src_lim"() -> (w917:dbl)
                n419 = call <instrlib>:"Configure Source Limit Level.vi"("error in (no error)"=w918, "Source Limit (1.0)"=w917, "Function (0: Volts)"=w916, "VISA resource name"=w919) -> ("error out"=w914:errorcluster, "VISA resource name out"=w915:refnum<visa-resource-name>)  [unwired: 6 in]
              }
              frame Enabled {
              }
            }
            n420 = local read "config_smu_funct"() -> (w908:u16)
            n421 = call <instrlib>:"Configure Measurement Function.vi"("error in (no error)"=w900, "Function (0: Volts)"=w908, "VISA resource name"=w901) -> ("error out"=w907:errorcluster)  [unwired: 7 in, 1 out]
          }
          frame Enabled {
            w933 = TRUE ("off_on")
            n422 = local read "current"() -> (w938:dbl)
            n423 = local read "vlim"() -> (w937:dbl)
            n424 = call "Set_Current_Meas_Res.vi"("vlim"=w937, "current"=w938, "VISA resource name"=w939) -> ("VISA resource name out"=w936:refnum<visa-resource-name>)  [unwired: 8 in]
            n425 = call "Set_Command.vi"("off_on"=w933, "command"=enum16{"Res_Sen", "Res_Comp"}."Res_Comp", "VISA resource name"=w936) -> ("VISA resource name out"=w934:refnum<visa-resource-name>)  [unwired: 7 in, 1 out]
            n426 = call "Set_Command.vi"("off_on"=w933, "command"=enum16{"Res_Sen", "Res_Comp"}."Res_Sen", "VISA resource name"=w934) -> ("error out"=w931:errorcluster)  [unwired: 7 in, 1 out]
          }
        }
      }
      event "set_cmnd": Value Change {
        n427 = event-data() -> ()  [unwired: 1 in, 1 out]
        n428 = Unbundle By Name(w946) -> ("smu_visa_res_out"=w943:refnum<visa-resource-name>)
        n429 = call "Set_Command.vi"("off_on"="off_on", "command"="command", "VISA resource name"=w943) -> ()  [unwired: 7 in, 2 out]
      }
      event "qry_cmd": Value Change {
        n430 = event-data() -> ()  [unwired: 1 in, 1 out]
        n431 = Unbundle By Name(w953) -> ("smu_visa_res_out"=w950:refnum<visa-resource-name>)
        n432 = call "Query_Command.vi"("command"="qry_cmd 2", "VISA resource name"=w950) -> ("resp"=→"resp":string)  [unwired: 8 in, 1 out]
      }
    }
    n433 = Unbundle By Name(w695) -> ("status"=w694:bool)
    n434 = Or(x=w694, y=w696) -> (x .or. y?=w687:bool)
  }
  n435 = Unregister For Events(event registration refnum=w18, error in=w17) -> (error out=w11:errorcluster)
  n436 = Release Queue(queue=w21, error in (no error)=w22) -> (error out=w12:errorcluster)  [unwired: 1 in, 2 out]
  n437 = Merge Errors(w11, w12, w13) -> (w15:errorcluster)
  n438 = Destroy User Event ("Destroy \nUser Event")(user event=w14, error in=w15) -> (error out=w16:errorcluster)
  n439 = disable-structure shown="Disabled" {
    disable-tunnel: w16 -> [w954 _]
    frame Disabled {
      n440 = call <vilib>:"Simple Error Handler.vi"("error in (no error)"=w954) -> ()  [unwired: 1 in, 8 out]
    }
    frame Enabled {
    }
  }
